vi "Process.vi"(8 "error in":errorcluster, 11 "Instrument.Example":refnum<class "Instrument.Oxford1820.lvclass">) -> (0 "error out":errorcluster, 3 "Instrument.Example out":refnum<class "Instrument.Oxford1820.lvclass">)   [LabVIEW 2019, in "Instrument.Oxford1820.lvclass"]
doc: "---------------------------------------------------------------\nJKI State Machine Objects™\nhttp://jki.net/state-machine-objects/\nCopyright (C) 2005-2015, JKI <info@jki.net>\nALL RIGHTS RESERVED"
uses:
  Instrument.Oxford1820.lvclass
  C:/Program Files/National Instruments/LabVIEW 2019/vi.lib/JKI/JKI SMO/SMO/SMO.lvclass
  C:/Program Files/National Instruments/LabVIEW 2019/user.lib/LevyLab/Instrument Framework/Instrument/Instrument.lvclass
  Typedefs/PrivateEvents--Instrument.Oxford1820.setMagnet.ctl
  <userlib>/LevyLab/Instrument Framework/Instrument Types/Cryostat/Typedefs/Magnet Axis--Enum.ctl
  <userlib>/LevyLab/Instrument Framework/Instrument Types/Cryostat/Typedefs/Magnet Mode--Enum.ctl
  <userlib>/LevyLab/Instrument Framework/Instrument Types/Cryostat/Typedefs/setMagnet--cluster.ctl
  <userlib>/LevyLab/RemoteControl/RemoteControl/Typedefs/Message--Cluster.ctl
  Typedefs/Instrument.Oxford1820.protectedCommands-enum.ctl
  Instrument.Oxford1820.lvclass/Instrument.Oxford1820.ctl
  <vilib>/JKI/JKI SMO/SMO/SMO.lvclass/SMO.ctl
  <instrlib>/Mercury iXX/Public/Libraries/Magnet/Controls/PSU Actions.ctl
  <instrlib>/Mercury iXX/Public/Libraries/Magnet/Controls/Switch Heater.ctl
  Typedefs/Fill Mode-Combo.ctl
  186db9c5-65d2-4fc6-8f89-8e5e62c6db85.vi
  d6eb67ea-c813-4959-b2d5-db01b126de05.vi
  79230e88-dac9-4f3c-b189-792686af81b5.vi
  2ec46187-1f5b-4c8a-9eba-53bd0c375d13.vi
  358ba730-dd62-46a8-9efd-e7dccbf66e54.vi
  c920ba95-1430-4558-8b27-62dbbfd83a50.vi
  <vilib>/dlg_ctls.llb/Space Constant.vi
  <vilib>/AdvancedString/1D String Array to Delimited String.vi
  186db9c5-65d2-4fc6-8f89-8e5e62c6db85.vi/0a7a26e5-3983-4de9-a886-1b2665f625f1.vi
  186db9c5-65d2-4fc6-8f89-8e5e62c6db85.vi/067870e1-bb36-4859-91df-debdbf4baae4.vi
  <vilib>/JKI/JKI SMO/SMO/Private/ReftoDVR--SMO.vi
  d6eb67ea-c813-4959-b2d5-db01b126de05.vi/35af6c41-d28b-4c86-bf85-588a84a7ed82.vi
  d6eb67ea-c813-4959-b2d5-db01b126de05.vi/18926865-8741-4660-bc11-64031fabb0ef.vi
  79230e88-dac9-4f3c-b189-792686af81b5.vi/9a2d704e-5f19-4206-ba54-236c9ffa4be8.vi
  79230e88-dac9-4f3c-b189-792686af81b5.vi/980f9c9d-13e7-4935-b9e6-1304dd0781c0.vi
  2ec46187-1f5b-4c8a-9eba-53bd0c375d13.vi/43f0deac-4eb7-47d7-baca-62a8f74b0a96.vi
  2ec46187-1f5b-4c8a-9eba-53bd0c375d13.vi/e6f40672-4e2f-465c-8f83-0c6010a026af.vi
  358ba730-dd62-46a8-9efd-e7dccbf66e54.vi/002d1415-4ace-441f-9214-6bf758fc91ec.vi
  358ba730-dd62-46a8-9efd-e7dccbf66e54.vi/d6bfcf14-f756-4c59-824c-a5b7ea6121ce.vi
  c920ba95-1430-4558-8b27-62dbbfd83a50.vi/42d7fbcc-e1e5-48c6-b631-238e61f5951c.vi
  c920ba95-1430-4558-8b27-62dbbfd83a50.vi/28ba82e0-a687-457f-9ef5-8b78e327060a.vi
  <vilib>/Utility/Data Type/Get Type Information.vi
  <vilib>/JDP Science/JSONtext/JSON text to Variant.vi
  <userlib>/LevyLab/Instrument Framework/Instrument/API/Instrument.sendMessageToProcess (variant).vi
  <vilib>/JDP Science/JSONtext/LVClass Serializer/JSONtext LVClass Serializer.lvclass
  <userlib>/LevyLab/Instrument Framework/Instrument Types/Cryostat/Instrument.Cryostat.lvclass
  <vilib>/JKI/JKI SMO/SMO/SMO.lvclass
  <instrlib>/Mercury iXX/Public/Libraries/Magnet.lvlib
  <userlib>/LevyLab/RemoteControl/RemoteControl/RemoteControl.lvclass
  <userlib>/LevyLab/Instrument Framework/Instrument/Instrument.lvclass
  <userlib>/LevyLab/Debug/Debug.lvlib
  C:/Program Files/National Instruments/LabVIEW 2019/user.lib/LevyLab/Instrument Framework/Instrument Types/Cryostat/Instrument.Cryostat.lvclass
panel:
  out "Timer":string
  out "State History":string
  out "timer":u32
  # "1820"
  # "1820"
  # "For instructions on how to use the JKI State Machine Objects, examples and video tutorials, visit:\nhttp://jki.net/state-machine-objects/\n\nJKI State Machine Objects™\nhttp://jki.net/state-machine-objects/\nCopyright (C) 2005-2015, JKI <info@jki.net>\nALL RIGHTS RESERVED"
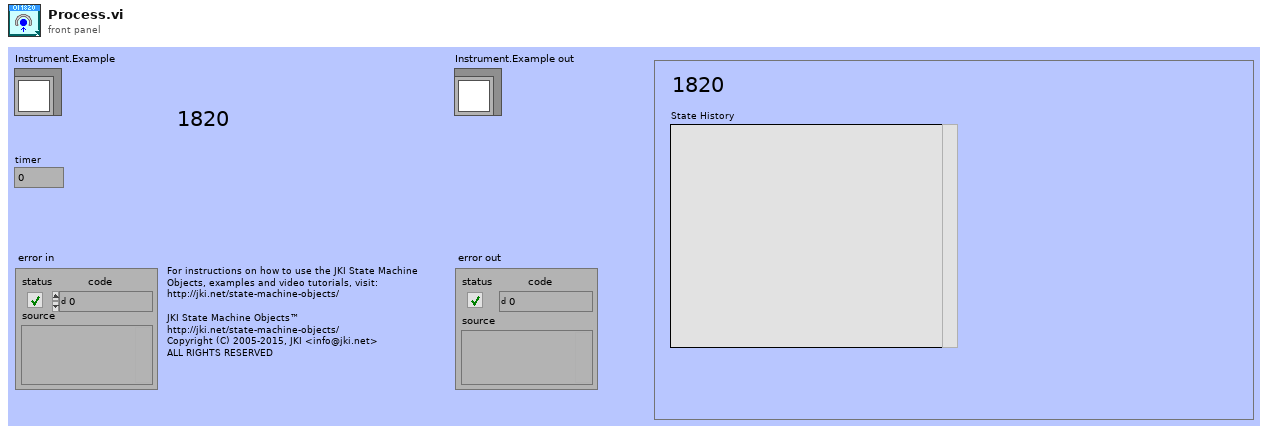
[diagram p1: front panel]
types:
  T1 = typedef "Instrument.Oxford1820.lvclass/PrivateEvents--Instrument.Oxford1820.setMagnet.ctl" = cluster{"field":dbl, "rate":dbl, "axis":T2, "mode":T3}
  T2 = typedef "Instrument.Cryostat.lvclass/Magnet Axis--Enum.ctl" = enum16{"X", "Y", "Z"}
  T3 = typedef "Instrument.Cryostat.lvclass/Magnet Mode--Enum.ctl" = enum16{"Persistent", "Driven"}
  T4 = typedef "Instrument.Cryostat.lvclass/setMagnet--cluster.ctl" = cluster{"field":dbl, "rate":dbl, "axis":T2, "mode":T3}
  T5 = enum32{"invalid app kind", "Development System", "Run Time System", "Student Edition", "Embedded LabVIEW", "Evaluation", "Custom"}
  T6 = typedef "RemoteControl.lvlib/RemoteControl.lvclass/Message--Cluster.ctl" = cluster{"Command":string, "Data":variant, "ID":string, "error":errorcluster}
  T7 = typedef "Instrument.Oxford1820.lvclass/Instrument.Oxford1820.protectedCommands-enum.ctl" = enum16{"Hold", "RampToSet", "RampToZero", "Clamp", "setTarget", "setSwitchHeat", "setLambda", "setFillMode", "setNeedleValve", "getStatus", "getTarget", "getSwitchHeat", "getPSUField", "setSequenceStatus"}
  T8 = enum32{"Invalid", "Standard", "Closed", "Hidden", "Minimized", "Maximized"}
  T9 = typedef "Mercury iXX.lvlib/Magnet.lvlib/PSU Actions.ctl" = string
  T10 = typedef "Mercury iXX.lvlib/Magnet.lvlib/Switch Heater.ctl" = string
  T11 = typedef "Instrument.Oxford1820.lvclass/Fill Mode-Combo.ctl" = string
  T12 = cluster{"Core":cluster{"Current VI Reference":refnum<vi>, "Close Panel on Exit?":bool, "Last Error":cluster{"error":errorcluster, "previous state":string, "remaining states":string}, "Shutdown?":bool}, "SMO":refnum<class "Instrument.Oxford1820.lvclass">, "setMagnet":T4, "Running Step":i32, "sequence":string[], "Message":T6}
  T13 = cluster{"Current VI Reference":refnum<vi>, "Close Panel on Exit?":bool, "Last Error":cluster{"error":errorcluster, "previous state":string, "remaining states":string}, "Shutdown?":bool}
  T14 = typedef "Debug.lvlib/Attribute.Debug.lvclass/DebugBehavior.ctl" = enum16{"Normal", "Debug"}
  T15 = typedef "SMO.lvclass/Protected Events.ctl" = cluster{"StopProcesses":refnum<user-event>, "AbortProcesses":refnum<user-event>, "Config Changed":refnum<user-event>, "Dependency":refnum<user-event>}
  T16 = typedef "Instrument.Oxford1820.lvclass/PrivateEvents--Cluster.ctl" = cluster{"SequenceSetMagnetField":refnum<user-event>, "AbortSequence":refnum<user-event>, "MessageToProcess":refnum<user-event>}
  T17 = typedef "Instrument.Oxford1820.lvclass/getAll.ctl" = cluster{"1820_IPS_Magnet_Field":dbl, "1820_IPS_PS_Field":dbl, "1820_IPS_Target_Field":dbl, "1820_IPS_Target_Field_Rate":dbl, "1820_IPS_Voltage":dbl, "1820_IPS_Current":dbl, "1820_IPS_Level_N2":dbl, "1820_IPS_Level_He":dbl, "1820_IPS_Magnet_Temperature":dbl, "1820_IPS_Magnet_Temperature_R":dbl, "1820_IPS_M1_Current":dbl, "1820_IPS_M1_Voltage":dbl, "1820_IPS_M2_Current":dbl, "1820_IPS_M2_Voltage":dbl, "1820_IPS_M3_Current":dbl, "1820_IPS_M3_Voltage":dbl, "1820_IPS_Status":string, "1820_IPS_Switch":string, "1820_ITC_Lambda_Temperature":dbl, "1820_ITC_Lambda_Temperature_R":dbl, "1820_ITC_Pressure":dbl, "1820_ITC_Needle_Valve":dbl}
  T18 = cluster{"Holding":bool, "Ramp to Setpoint":bool, "Ramp to Zero":bool, "Clamp":bool}
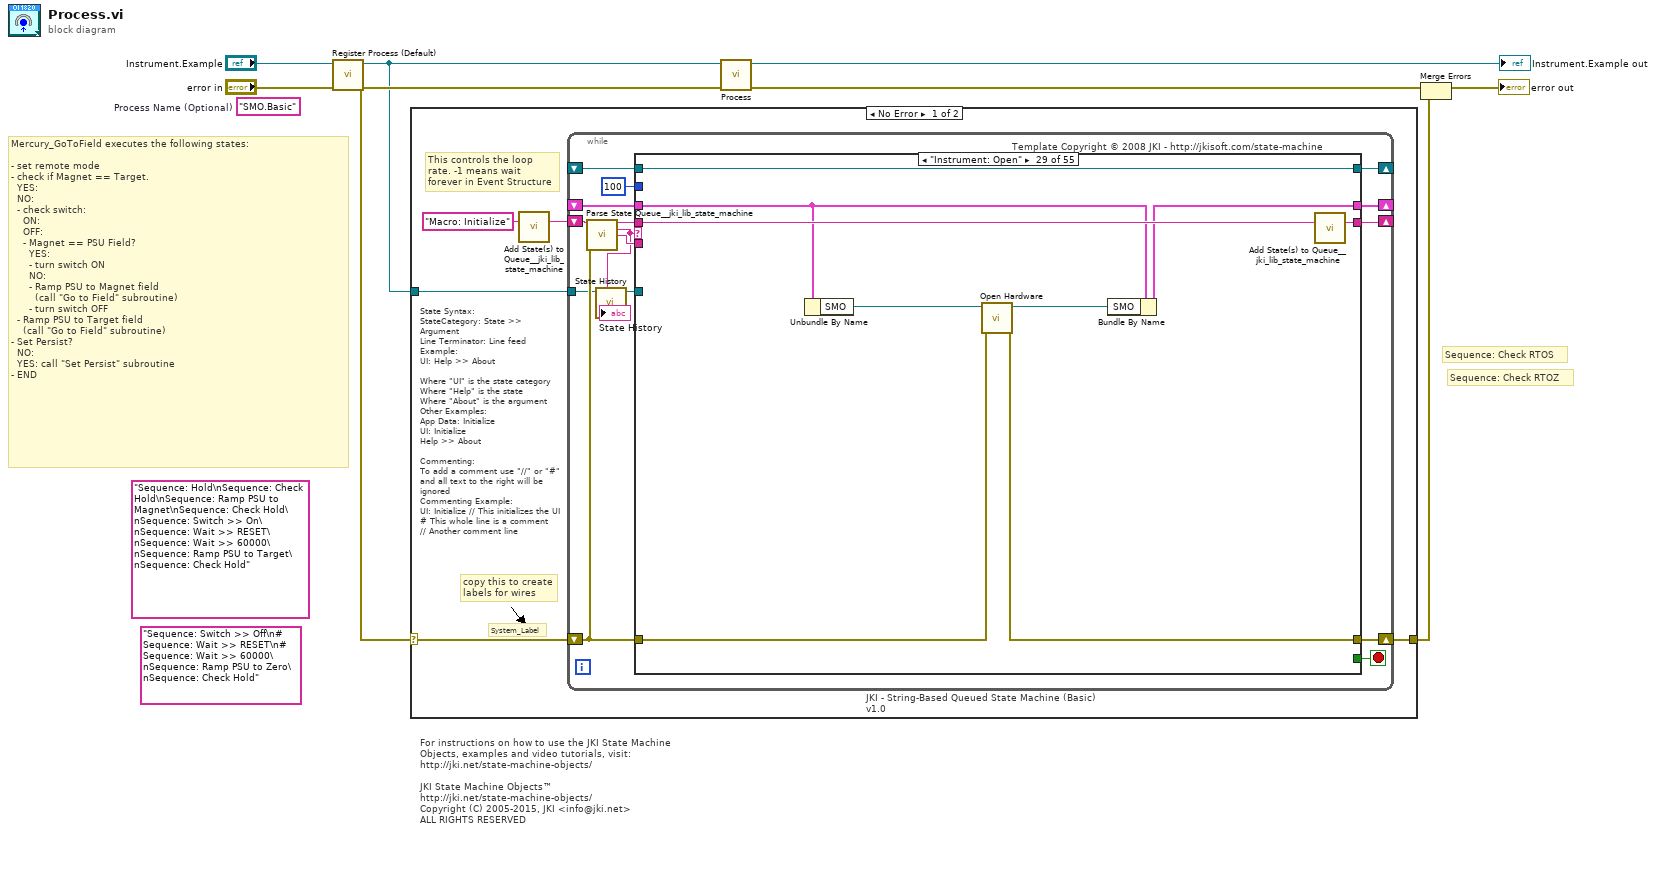
[diagram p0: block diagram]
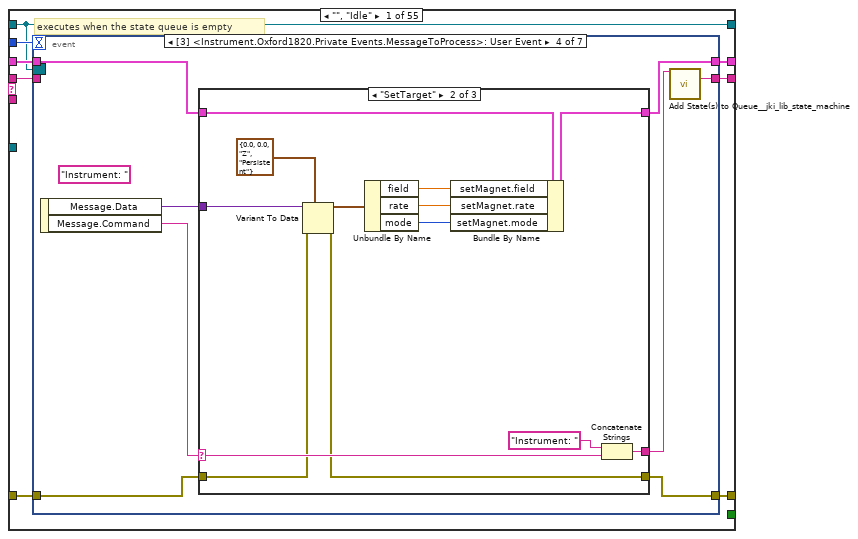
[diagram p2: hidden frame]
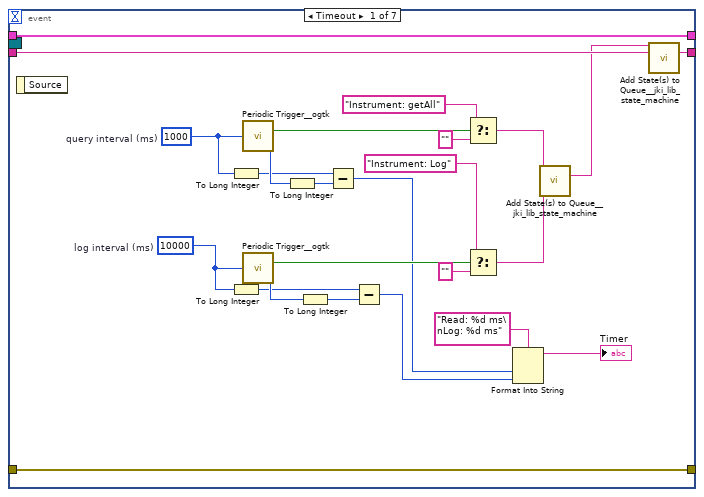
[diagram p3: hidden frame]
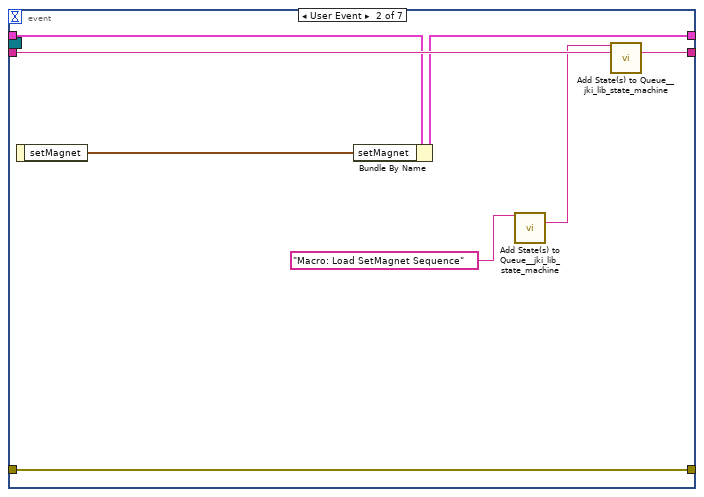
[diagram p4: hidden frame]
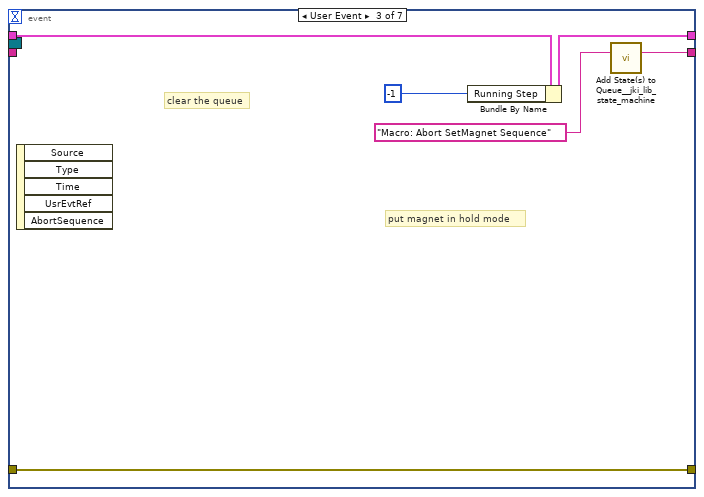
[diagram p5: hidden frame]
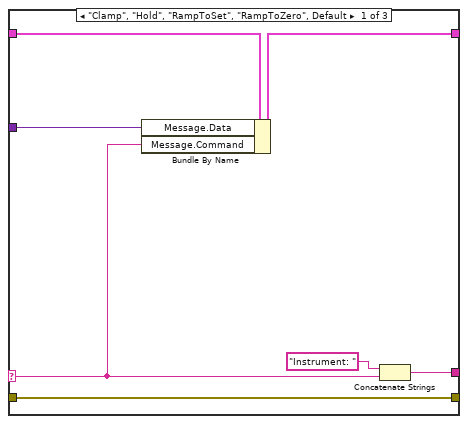
[diagram p6: hidden frame]
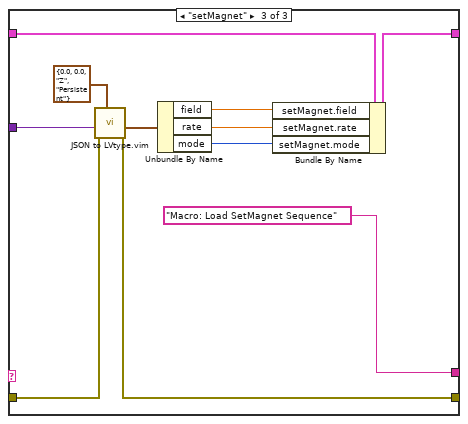
[diagram p7: hidden frame]
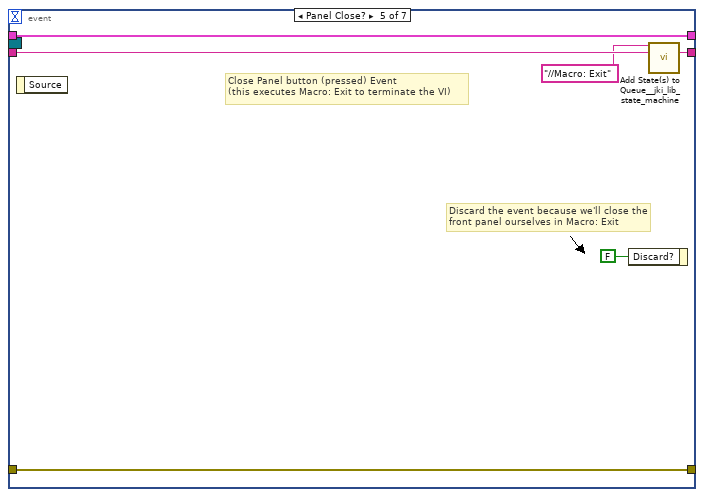
[diagram p8: hidden frame]
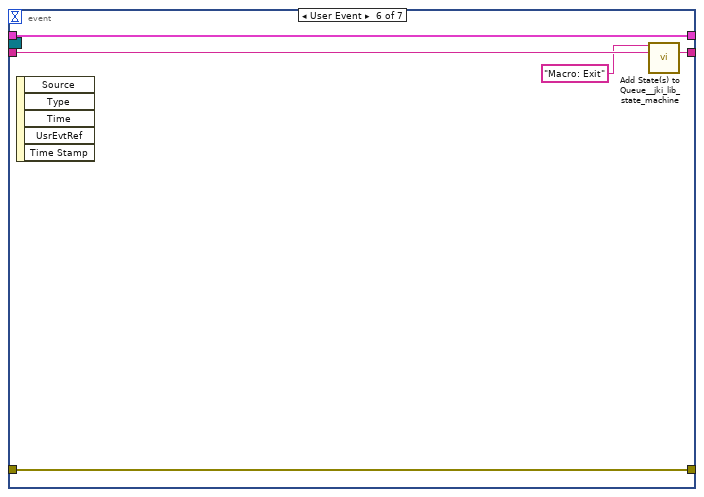
[diagram p9: hidden frame]
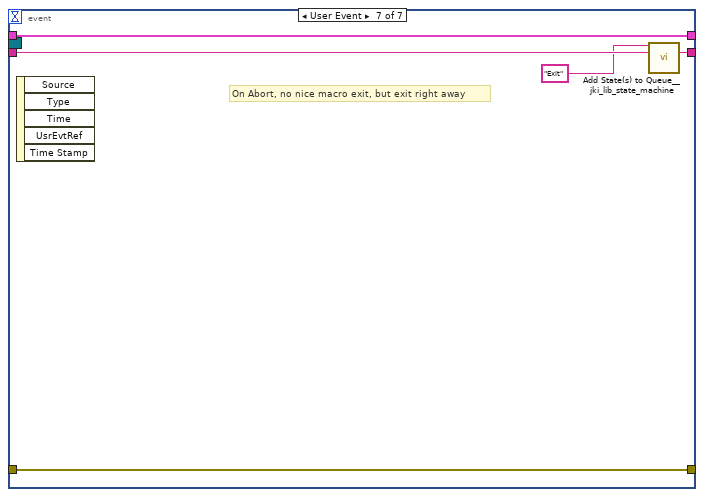
[diagram p10: hidden frame]
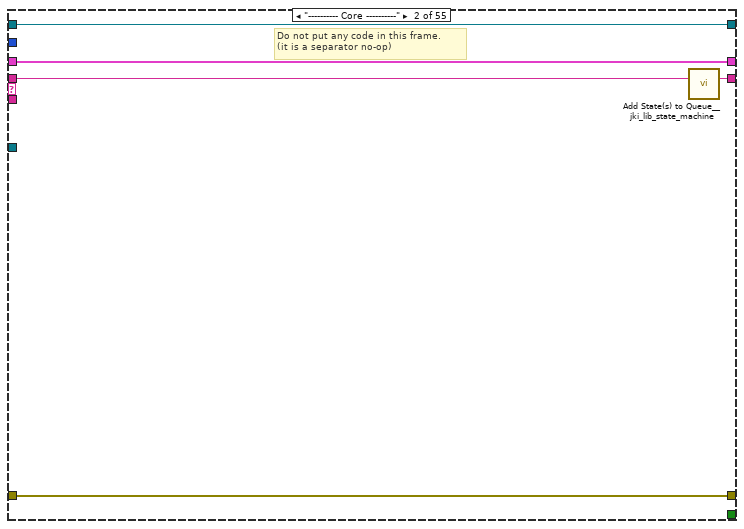
[diagram p11: hidden frame]
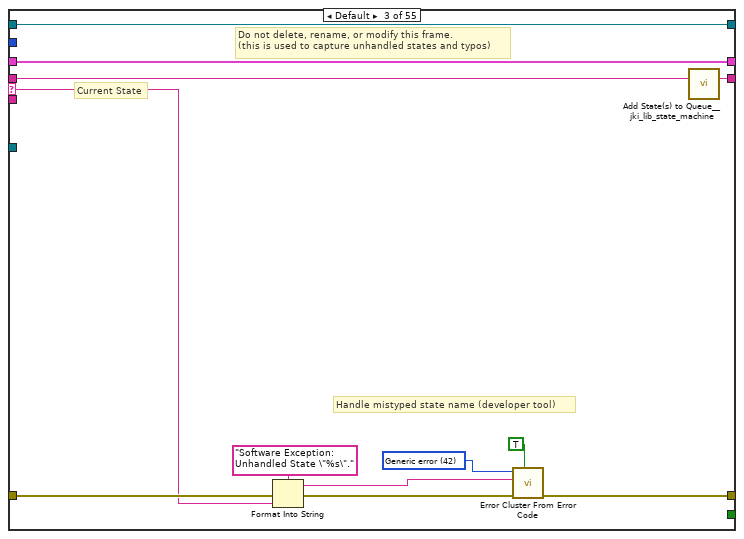
[diagram p12: hidden frame]
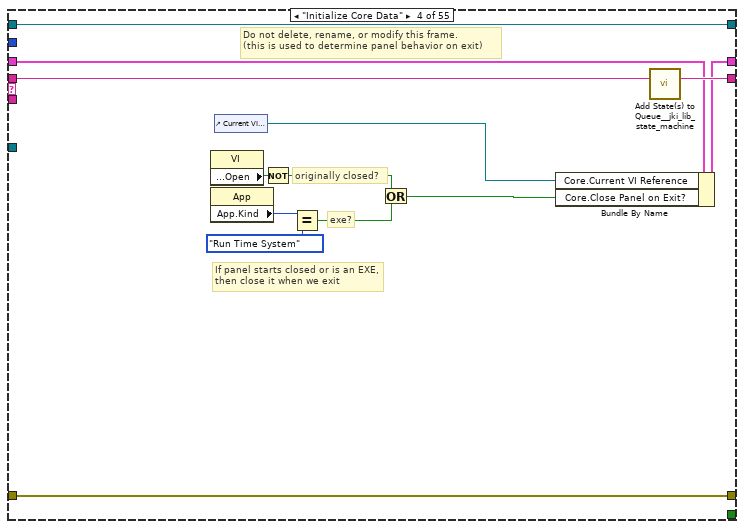
[diagram p13: hidden frame]
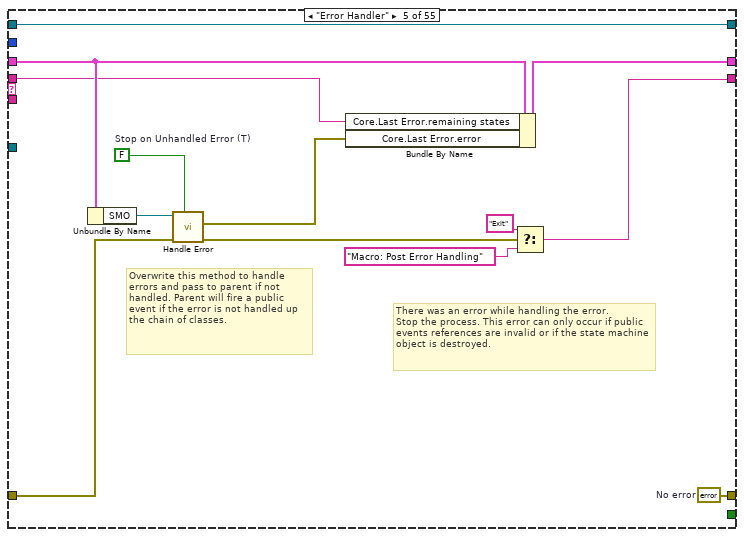
[diagram p14: hidden frame]
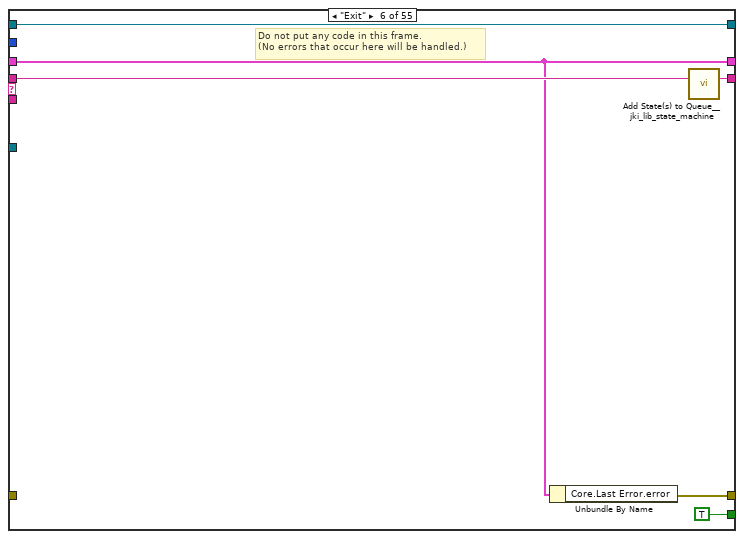
[diagram p15: hidden frame]
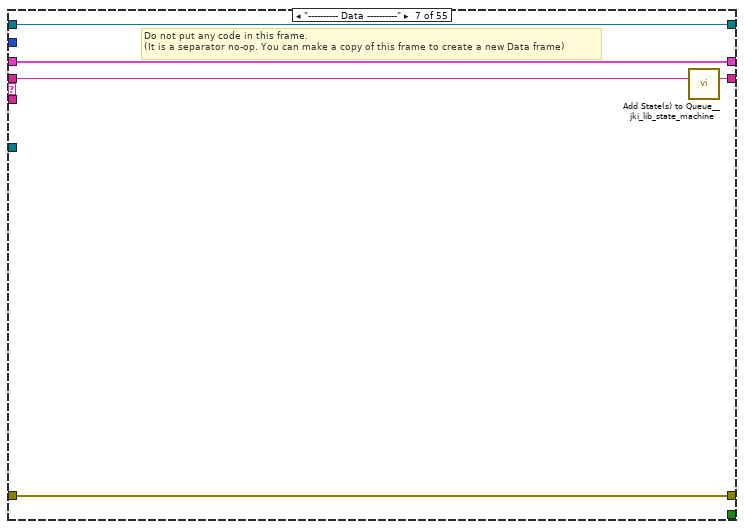
[diagram p16: hidden frame]
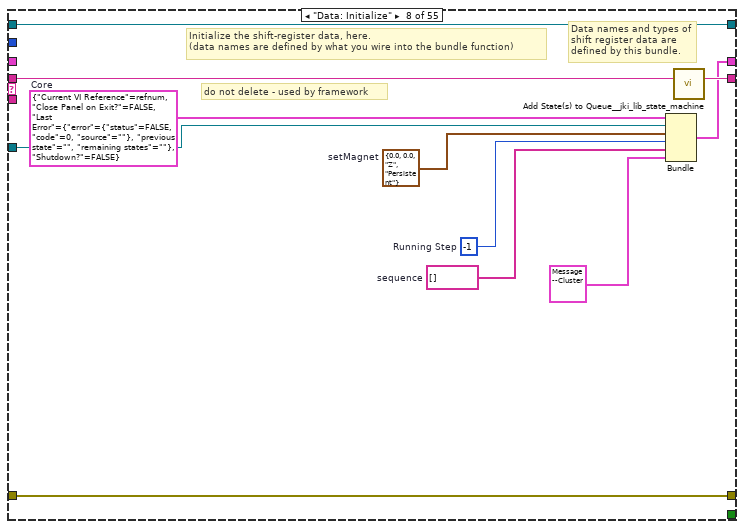
[diagram p17: hidden frame]
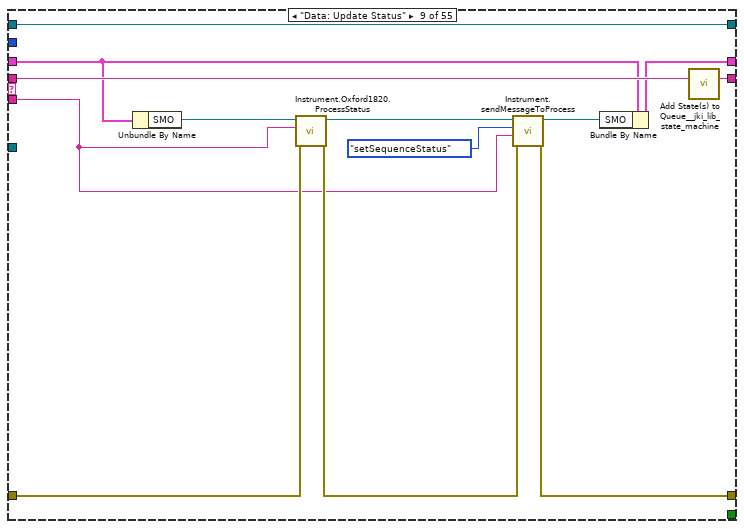
[diagram p18: hidden frame]
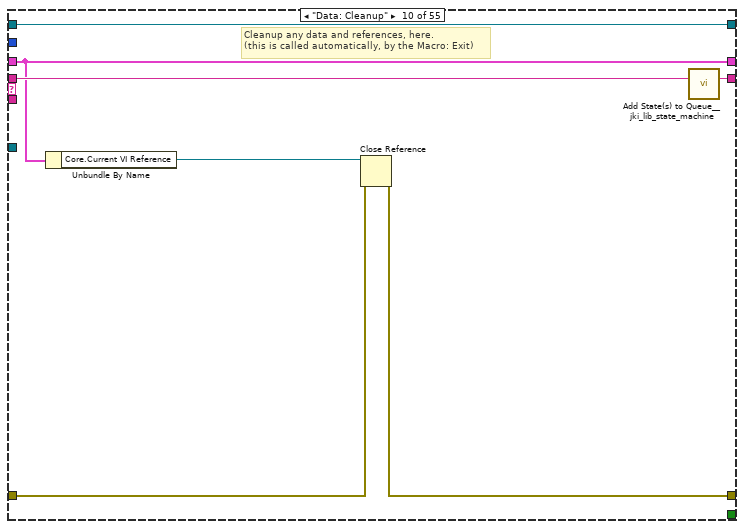
[diagram p19: hidden frame]
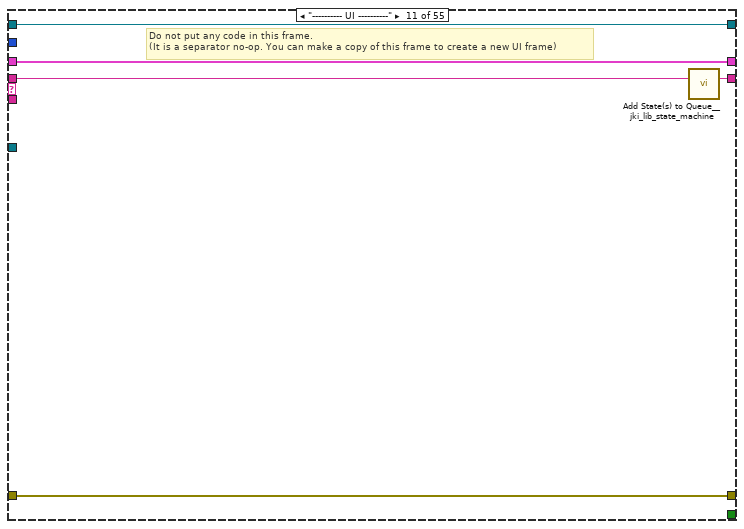
[diagram p20: hidden frame]
diagram:
  (unwired) "Sequence: Switch >> Off\n# Sequence: Wait >> RESET\n# Sequence: Wait >> 60000\nSequence: Ramp PSU to Zero\nSequence: Check Hold" ("State(s) in Front (\"\")")
  (unwired) "Sequence: Hold\nSequence: Check Hold\nSequence: Ramp PSU to Magnet\nSequence: Check Hold\nSequence: Switch >> On\nSequence: Wait >> RESET\nSequence: Wait >> 60000\nSequence: Ramp PSU to Target\nSequence: Check Hold" ("State(s) in Front (\"\")")
  (unwired) "SMO.Basic"  # Process Name (Optional)
  # "Sequence: Check RTOZ"
  # "Sequence: Check RTOS"
  # "Mercury_GoToField executes the following states:\n\n- set remote mode\n- check if Magnet == Target.\n  YES:\n  NO:\n  - check switch:\n    ON:\n    OFF:\n    - Magnet == PSU Field?\n      YES:\n      - turn switch ON\n      NO:\n      - Ramp PSU to Magnet field\n        (call \"Go to Field\" subroutine)\n      - turn switch OFF\n  - Ramp PSU to Target field\n    (call \"Go to Field\" subroutine)\n- Set Persist?\n  NO:\n  YES: call \"Set Persist\" subroutine\n- END"
  # "For instructions on how to use the JKI State Machine Objects, examples and video tutorials, visit:\nhttp://jki.net/state-machine-objects/\n\nJKI State Machine Objects™\nhttp://jki.net/state-machine-objects/\nCopyright (C) 2005-2015, JKI <info@jki.net>\nALL RIGHTS RESERVED"
  n1 = call <vilib>:"Register Process (Default).vi"("error in (no error)"="error in", "SMO"="Instrument.Example") -> ("error out"=w5:errorcluster, "SelfRef"=w4:refnum<class "Instrument.Oxford1820.lvclass">)  [unwired: 8 in]
  n2 = case shown="No Error" w5 {
    selector: w5 -> [w10 w914]
    tunnel: w4 -> [w11 _]
    tunnel: [w9 w914] -> w1
    frame No Error {
      # "State Syntax:\nStateCategory: State >> Argument\nLine Terminator: Line feed\nExample:\nUI: Help >> About\n\nWhere \"UI\" is the state category\nWhere \"Help\" is the state\nWhere \"About\" is the argument\nOther Examples:\nApp Data: Initialize\nUI: Initialize\nHelp >> About\n\nCommenting:\nTo add a comment use \"//\" or \"#\" and all text to the right will be ignored\nCommenting Example:\nUI: Initialize // This initializes the UI\n# This whole line is a comment\n// Another comment line"
      # "copy this to create labels for wires"
      # "This controls the loop rate. -1 means wait forever in Event Structure"
      # "System_Label"
      n3 = call <vilib>:"Add State(s) to Queue__jki_lib_state_machine.vi"("State(s) in (\"\")"="Macro: Initialize") -> ("States Out"=w13:string)  [unwired: 14 in]
      n4 = while "JKI - String-Based Queued State Machine (Basic) v1.0" {
        shift-right: [w23] -> _
        shift-left: _ -> [w22]
        shift-right: [w26] -> w9
        shift-left: w10 -> [w20]
        shift-right: [w25] -> _
        shift-left: w13 -> [w27]
        tunnel: w11 -> [w14]
        shift-right: [w19] -> _
        shift-left: _ -> [w18]
        stop <- w24 stop-if-true
        # "Template Copyright © 2008 JKI - http://jkisoft.com/state-machine"
        n5 = call <vilib>:"Parse State Queue__jki_lib_state_machine.vi"("State Queue"=w27, "Error In (no error)"=w20) -> ("Remaining States"=w29:string, "Current State"=w16:string, "Arguments"=w28:string)  [unwired: 11 in]
        n6 = call <userlib>:"State History.vi"("Current State"=w16, "SMO"=w14) -> ("SMO"=w15:refnum<class "Instrument.Oxford1820.lvclass">, "History"=→"State History":string)  [unwired: 8 in]
        n7 = case shown="\"Instrument: Open\"" w16 {
          selector: w16 -> [_ _ w138 _ _ _ _ _ _ _ _ _ _ _ _ _ _ _ _ _ _ _ _ _ _ _ _ _ _ _ _ _ _ _ _ _ _ _ _ _ _ _ _ _ _ w687 w711 w744 w776 w797 w817 w837 w858 w877 w904]
          tunnel: w29 -> [w37 w136 w142 w161 w163 w180 w185 w196 w209 w216 w221 w228 w235 w251 w283 w292 w309 w324 w346 w349 _ _ w405 w416 w421 w434 w440 w447 w456 w465 w477 w490 w503 w520 w533 w550 w560 w573 w598 w618 w631 w644 w653 w662 w684 w696 w717 w750 w782 w804 w825 w846 w867 w888 w913]
          tunnel: w28 -> [_ _ _ _ _ _ _ _ w197 _ _ _ w229 w245 _ _ _ _ _ _ _ _ _ _ _ _ _ _ _ _ _ _ w493 _ _ _ _ w565 w584 _ _ _ _ _ w668 _ w710 _ _ _ _ _ _ _ _]
          tunnel: w22 -> [w35 w133 w140 w152 w170 w176 w182 _ w206 w211 w218 w226 w233 w247 w280 w289 w293 w311 w335 w350 w366 w393 w402 w413 w418 w432 w438 w442 w452 w461 w474 w487 w496 w515 w526 w545 w555 w562 w594 w614 w627 w640 w649 w656 w671 w693 w714 w746 w779 w801 w819 w840 w861 w885 w910]
          tunnel: [w34 w134 w144 w158 w171 w175 w183 w187 w198 w212 w219 w222 w230 w248 w281 w284 w307 w314 w344 w351 w367 w391 w403 w407 w419 w427 w436 w444 w448 w457 w467 w478 w491 w511 w527 w542 w551 w563 w588 w608 w622 w637 w647 w659 w672 w689 w698 w735 w769 w795 w811 w831 w852 w872 w903] -> w26
          tunnel: w20 -> [w33 w134 w143 w158 w172 _ w183 w187 w204 w213 w219 w223 w231 w249 w281 w284 w307 w313 w344 w351 w367 w391 w403 w408 w419 w428 w436 w444 w449 w458 w472 w479 w494 w513 w525 w543 w553 w566 w585 w606 w619 w633 w646 w659 w669 w689 w697 w734 w768 w795 w805 w826 w847 w868 w889]
          tunnel: [w36 w135 w141 w160 w162 w179 w184 w195 w208 w215 w220 w227 w234 w250 w282 w291 w308 w323 w345 w348 w383 w400 w404 w415 w420 w433 w439 w446 w455 w464 w476 w489 w502 w519 w532 w549 w559 w572 w597 w617 w630 w643 w652 w661 w683 w695 w716 w749 w781 w803 w824 w845 w866 w887 w912] -> w25
          tunnel: [_ _ _ _ _ TRUE _ _ _ _ _ _ _ _ _ _ _ _ _ _ _ _ _ _ _ _ _ _ _ _ _ _ _ _ _ _ _ _ _ _ _ _ _ _ _ _ _ _ _ _ _ _ _ _ _] -> w24
          tunnel: [w32 w133 w140 w159 w169 w176 w182 w194 w203 w211 w218 w226 w233 w247 w280 w289 w294 w312 w342 w347 w375 w395 w402 w413 w418 w432 w438 w441 w450 w459 w473 w486 w500 w517 w530 w547 w557 w570 w595 w615 w628 w641 w650 w655 w665 w692 w713 w745 w778 w800 w818 w839 w860 w884 w909] -> w23
          tunnel: 100 ("Timeout") -> [w31 _ _ _ _ _ _ _ _ _ _ _ _ _ _ _ _ _ _ _ _ _ _ _ _ _ _ _ _ _ _ _ _ _ _ _ _ _ _ _ _ _ _ _ _ _ _ _ _ _ _ _ _ _ _]
          tunnel: w15 -> [_ _ _ _ _ _ _ w188 _ _ _ _ _ _ _ _ _ _ _ _ _ _ _ _ _ _ _ _ _ _ _ _ _ _ _ _ _ _ _ _ _ _ _ _ _ _ _ _ _ _ _ _ _ _ _]
          tunnel: [w30 w132 w137 w149 w174 w177 w181 w193 w207 w210 w217 w225 w232 w244 w279 w290 w301 w322 w343 w358 w382 w399 w401 w414 w417 w431 w437 w445 w454 w463 w475 w488 w501 w518 w531 w548 w558 w571 w596 w616 w629 w642 w651 w660 w682 w694 w715 w748 w780 w802 w823 w844 w865 w886 w911] -> w19
          tunnel: w18 -> [w30 w132 w137 w149 w174 w177 w181 w193 w207 w210 w217 w225 w232 w244 w279 w290 w301 w322 w343 w358 w382 w399 w401 w414 w417 _ w437 w445 w454 w463 w475 w488 w501 w518 w531 w548 w558 w571 w596 w616 w629 w642 w651 w660 w682 w694 w715 w748 w780 w802 w823 w844 w865 w886 w911]
          frame "", "Idle" {
            # "executes when the state queue is empty"
            n8 = event shown="[3] <Instrument.Oxford1820.Private Events.MessageToProcess>: User Event" {
              selector: w30 -> [_ _ _ _ _ _ _]
              dyn-events: _ -> [_ _ _ _ _ _ _]
              timeout: w31 -> [_ _ _ _ _ _ _]
              tunnel: w37 -> [w62 w68 _ _ w121 w126 w131]
              tunnel: [w61 w69 w75 w84 w120 w125 w130] -> w36
              tunnel: w35 -> [w59 w67 w73 w79 w118 w123 w128]
              tunnel: [w60 w70 w76 w83 w119 w124 w129] -> w34
              tunnel: w33 -> [w60 w70 w76 w82 w119 w124 w129]
              tunnel: [w59 w66 w72 w78 w118 w123 w128] -> w32
              event Timeout {
                w38 = u32 10000  # log interval (ms)
                w39 = u32 1000  # query interval (ms)
                n9 = event-data() -> ()  [unwired: 1 in, 1 out]
                n10 = To Long Integer(number=w39) -> (32bit integer=w45:i32)
                n11 = To Long Integer(number=w38) -> (32bit integer=w46:i32)
                n12 = call <userlib>:"Periodic Trigger__ogtk.vi"("time (ms)"=w39) -> ("Triggered"=w58:bool, "timer value"=w52:u32)  [unwired: 12 in, 1 out]
                n13 = call <userlib>:"Periodic Trigger__ogtk.vi"("time (ms)"=w38) -> ("Triggered"=w55:bool, "timer value"=w51:u32)  [unwired: 12 in, 1 out]
                n14 = To Long Integer(number=w52) -> (32bit integer=w44:i32)
                n15 = To Long Integer(number=w51) -> (32bit integer=w43:i32)
                n16 = Subtract(x=w45, y=w44) -> (x-y=w50:i32)
                n17 = Subtract(x=w46, y=w43) -> (x-y=w49:i32)
                n18 = Select(t="Instrument: getAll", s=w58, f="") -> (s? t:f=w53:string)
                n19 = Select(t="Instrument: Log", s=w55, f="") -> (s? t:f=w54:string)
                n20 = Format Into String(format string="Read: %d ms\nLog: %d ms", w50, w49) -> (resulting string=→"Timer":string)  [unwired: 2 in, 1 out]
                n21 = call <vilib>:"Add State(s) to Queue__jki_lib_state_machine.vi"("State(s) in Front (\"\")"=w53, "State(s) at Back (\"\")"=w54) -> ("States Out"=w40:string)  [unwired: 13 in]
                n22 = call <vilib>:"Add State(s) to Queue__jki_lib_state_machine.vi"("State(s) in Front (\"\")"=w40, "State(s) in (\"\")"=w62) -> ("States Out"=w61:string)  [unwired: 13 in]
              }
              event User Event {
                n23 = event-data() -> ("setMagnet"=w63:T4)  [unwired: 1 in]
                n24 = Bundle By Name(cluster=w67, "setMagnet"=w63) -> (w66:T12)
                n25 = call <vilib>:"Add State(s) to Queue__jki_lib_state_machine.vi"("State(s) in Front (\"\")"="Macro: Load SetMagnet Sequence" ("State(s) at Back (\"\")")) -> ("States Out"=w64:string)  [unwired: 14 in]
                n26 = call <vilib>:"Add State(s) to Queue__jki_lib_state_machine.vi"("State(s) in Front (\"\")"=w64, "State(s) in (\"\")"=w68) -> ("States Out"=w69:string)  [unwired: 13 in]
              }
              event User Event {
                # "put magnet in hold mode"
                # "clear the queue"
                n27 = event-data() -> ()  [unwired: 1 in, 5 out]
                n28 = Bundle By Name(cluster=w73, "Running Step"=-1) -> (w72:T12)
                n29 = call <vilib>:"Add State(s) to Queue__jki_lib_state_machine.vi"("State(s) in (\"\")"="Macro: Abort SetMagnet Sequence" ("State(s) at Back (\"\")")) -> ("States Out"=w75:string)  [unwired: 14 in]
              }
              event User Event {
                (unwired) "Instrument: " ("State(s) at Back (\"\")")
                n30 = event-data() -> ("Message.Data"=w80:variant, "Message.Command"=w81:string)  [unwired: 1 in]
                n31 = case shown="\"SetTarget\"" w81 {
                  selector: w81 -> [w87 w103 _]
                  tunnel: w79 -> [w85 w101 w115]
                  tunnel: [w86 w100 w114] -> w78
                  tunnel: [w91 w104 "Macro: Load SetMagnet Sequence" ("State(s) at Back (\"\")")] -> w77
                  tunnel: w80 -> [w88 w99 w109]
                  tunnel: w82 -> [w89 w97 w106]
                  tunnel: [w89 w96 w105] -> w83
                  frame "Clamp", "Hold", "RampToSet", "RampToZero", Default {
                    n32 = Bundle By Name(cluster=w85, "Message.Data"=w88, "Message.Command"=w87) -> (w86:T12)
                    n33 = Concatenate Strings("Instrument: " ("State"), w87) -> (w91:string)
                  }
                  frame "SetTarget" {
                    n34 = Variant To Data(error in=w97, type=T1 {"field"=0.0, "rate"=0.0, "axis"=enum."Z", "mode"=enum."Persistent"} ("Set Magnet Field"), Variant=w99) -> (data=w95:T1, error out=w96:errorcluster)
                    n35 = Unbundle By Name(w95) -> ("field"=w94:dbl, "rate"=w98:dbl, "mode"=w92:T3)
                    n36 = Bundle By Name(cluster=w101, "setMagnet.field"=w94, "setMagnet.rate"=w98, "setMagnet.mode"=w92) -> (w100:T12)
                    n37 = Concatenate Strings("Instrument: " ("State"), w103) -> (w104:string)
                  }
                  frame "setMagnet" {
                    n38 = call "JSON to LVtype.vim"("type"=T4 {"field"=0.0, "rate"=0.0, "axis"=enum."Z", "mode"=enum."Persistent"} ("setMagnet"), "error in (no error)"=w106, "JSON Data in"=w109) -> ("error out"=w105:errorcluster, "Data out"=w107:T4)  [unwired: 7 in]
                    n39 = Unbundle By Name(w107) -> ("field"=w110:dbl, "rate"=w111:dbl, "mode"=w112:T3)
                    n40 = Bundle By Name(cluster=w115, "setMagnet.field"=w110, "setMagnet.rate"=w111, "setMagnet.mode"=w112) -> (w114:T12)
                  }
                }
                n41 = call <vilib>:"Add State(s) to Queue__jki_lib_state_machine.vi"("State(s) in Front (\"\")"=w77) -> ("States Out"=w84:string)  [unwired: 14 in]
              }
              event Panel Close? {
                # "Discard the event because we'll close the front panel ourselves in Macro: Exit"
                # "Close Panel button (pressed) Event\n(this executes Macro: Exit to terminate the VI)"
                n42 = event-data() -> ()  [unwired: 1 in, 1 out]
                n43 = event-data("Discard?"=FALSE) -> ()  [unwired: 1 in, 1 out]
                n44 = call <vilib>:"Add State(s) to Queue__jki_lib_state_machine.vi"("State(s) in Front (\"\")"="//Macro: Exit", "State(s) in (\"\")"=w121) -> ("States Out"=w120:string)  [unwired: 13 in]
              }
              event User Event {
                n45 = event-data() -> ()  [unwired: 1 in, 5 out]
                n46 = call <vilib>:"Add State(s) to Queue__jki_lib_state_machine.vi"("State(s) in Front (\"\")"="Macro: Exit", "State(s) in (\"\")"=w126) -> ("States Out"=w125:string)  [unwired: 13 in]
              }
              event User Event {
                # "On Abort, no nice macro exit, but exit right away"
                n47 = event-data() -> ()  [unwired: 1 in, 5 out]
                n48 = call <vilib>:"Add State(s) to Queue__jki_lib_state_machine.vi"("State(s) in Front (\"\")"="Exit", "State(s) in (\"\")"=w131) -> ("States Out"=w130:string)  [unwired: 13 in]
              }
            }
          }
          frame "---------- Core ----------" {
            # "Do not put any code in this frame.\n(it is a separator no-op)"
            n49 = call <vilib>:"Add State(s) to Queue__jki_lib_state_machine.vi"("State(s) in (\"\")"=w136) -> ("States Out"=w135:string)  [unwired: 14 in]
          }
          frame Default {
            w147 = 42 items=["No error", "Argument error", "Memory is full", "Out of zone", "End of file", "File already open", "Generic file I/O error", "File not found", "File permission error", "Disk is full", "Duplicate path", "Too many files open", "System feature not enabled", "Resource file not found", "Cannot add resource", "Resource not found", "Image not found", "Image memory error", "Pen does not exist", "Config type invalid", "Config token not found", "Config parse error", "Config memory error", "Bad external code format", "Bad external code offset", "External code not present", "Null window", "Destroy window error", "Null menu", "Print aborted", "Bad print record", "Print driver error", "Windows error during printing", "Memory error during printing", "Print dialog error", "Generic print error", "Invalid device refnum", "Device not found", "Device parameter error", "Device unit error", "Cannot open device", "Device call aborted", "Generic error", "Cancelled by user", "Object ID too low", "Object ID too high", "Object not in heap", "Unknown heap", "Unknown object (invalid DefProc)", "Unknown object (DefProc not in table)", "Message out of range", "Invalid (null) method", "Unknown message", "Manager call not supported", "Bad address", "Network operation in progress", "Network operation timed out", "Connection is busy", "Network attribute not supported", "Network error", "Address in use", "System out of memory", "Connection aborted", "Connection refused", "Not connected", "Already connected", "Connection closed", "Initialization error (interapplication manager)", "Bad occurrence", "Wait on unbound occurrence handler", "Occurrence queue overflow", "Datalog type conflict", "Unused", "Unrecognized type (interapplication manager)", "Memory corrupt", "Failed to make temporary DLL", "Old CIN version", "Drag socket not found", "Failed to load drop-object", "Failed to register OLE object", "Failed to release OLE object", "Format specifier type mismatch", "Unknown format specifier", "Too few format specifiers", "Too many format specifiers", "Scan failed", "Newer CIN version", "Error converting to variant", "Runtime menu error", "Password tampered", "Variant attribute not found", "Incompatible variant data type", "Event data is not available", "Event Store is not present", "Occurrence is not found", "Event Queue is not created", "Event info is not available", "Refnum passed is NULL", "Error retrieving Class GUID", "Error retrieving CoClass GUID", "Error retrieving TypeLib GUID.", "Bad built application magic bytes.", "Specific driver is different from the specific driver associated with the Logical Name.", "There is no session opened to the class driver.", "Max Error", "MAX - Error with config objects", "MAX - Error loading configuration", "MAX - Group not supported"]
            # "Current State"
            # "Do not delete, rename, or modify this frame.\n(this is used to capture unhandled states and typos)"
            # "Handle mistyped state name (developer tool)"
            n50 = Format Into String(format string="Software Exception: Unhandled State \"%s\"." ("message"), error in=w143, w138) -> (resulting string=w146:string, error out=w145:errorcluster)  [unwired: 1 in]
            n51 = call <vilib>:"Error Cluster From Error Code.vi"("show call chain? (False)"=TRUE, "error in (no error)"=w145, "error message (\"\")"=w146, "error code (0)"=w147) -> ("error out"=w144:errorcluster)  [unwired: 5 in]
            n52 = call <vilib>:"Add State(s) to Queue__jki_lib_state_machine.vi"("State(s) in (\"\")"=w142) -> ("States Out"=w141:string)  [unwired: 14 in]
          }
          frame "Initialize Core Data" {
            # "Do not delete, rename, or modify this frame.\n(this is used to determine panel behavior on exit)"
            # "originally closed?"
            # "exe?"
            # "If panel starts closed or is an EXE, then close it when we exit"
            n53 = property class="VI"() -> ("Front Panel.Open"=w157:bool)  [unwired: 2 in, 2 out]
            n54 = property class="App"() -> ("App.Kind"=w156:T5)  [unwired: 2 in, 2 out]
            n55 = control-ref of="Current VI Reference"() -> (w150:refnum<vi>)
            n56 = Not(x=w157) -> (.not. x?=w154:bool)
            n57 = Equal?(x=w156, y=T5."Run Time System" ("Application:Kind")) -> (x = y?=w153:bool)
            n58 = Or(x=w154, y=w153) -> (x .or. y?=w151:bool)
            n59 = Bundle By Name(cluster=w152, "Core.Current VI Reference"=w150, "Core.Close Panel on Exit?"=w151) -> (w159:T12)
            n60 = call <vilib>:"Add State(s) to Queue__jki_lib_state_machine.vi"("State(s) in (\"\")"=w161) -> ("States Out"=w160:string)  [unwired: 14 in]
          }
          frame "Error Handler" {
            w165 = FALSE  # Stop on Unhandled Error (T)
            w171 = errorcluster {"status"=FALSE, "code"=0, "source"=""}  # No error
            # "There was an error while handling the error.\nStop the process. This error can only occur if public events references are invalid or if the state machine object is destroyed."
            # "Overwrite this method to handle errors and pass to parent if not handled. Parent will fire a public event if the error is not handled up the chain of classes."
            n61 = Unbundle By Name(w170) -> ("SMO"=w173:refnum<class "Instrument.Oxford1820.lvclass">)
            n62 = call-dynamic "Handle Error.vi"("Stop on Unhandled Error (T)"=w165, "error in"=w172, "SMO"=w173) -> ("handling error"=w166:errorcluster, "Unhandled error"=w168:errorcluster)  [unwired: 6 in, 1 out]
            n63 = Bundle By Name(cluster=w170, "Core.Last Error.remaining states"=w163, "Core.Last Error.error"=w168) -> (w169:T12)
            n64 = Select(t="Exit", s=w166, f="Macro: Post Error Handling") -> (s? t:f=w162:string)
          }
          frame "Exit" {
            # "Do not put any code in this frame.\n(No errors that occur here will be handled.)"
            n65 = Unbundle By Name(w176) -> ("Core.Last Error.error"=w175:errorcluster)
            n66 = call <vilib>:"Add State(s) to Queue__jki_lib_state_machine.vi"("State(s) in (\"\")"=w180) -> ("States Out"=w179:string)  [unwired: 14 in]
          }
          frame "---------- Data ----------" {
            # "Do not put any code in this frame.\n(It is a separator no-op. You can make a copy of this frame to create a new Data frame)"
            n67 = call <vilib>:"Add State(s) to Queue__jki_lib_state_machine.vi"("State(s) in (\"\")"=w185) -> ("States Out"=w184:string)  [unwired: 14 in]
          }
          frame "Data: Initialize" {
            w186 = T4 {"field"=0.0, "rate"=0.0, "axis"=enum."Z", "mode"=enum."Persistent"}  # setMagnet
            w190 = string[] []  # sequence
            w191 = -1  # Running Step
            w192 = T13 {"Current VI Reference"=refnum, "Close Panel on Exit?"=FALSE, "Last Error"={"error"={"status"=FALSE, "code"=0, "source"=""}, "previous state"="", "remaining states"=""}, "Shutdown?"=FALSE}  # Core
            # "do not delete - used by framework"
            # "Data names and types of shift register data are defined by this bundle."
            # "Initialize the shift-register data, here.\n(data names are defined by what you wire into the bundle function)"
            n68 = Bundle("Core"=w192, "SMO"=w188, "setMagnet"=w186, "Running Step"=w191, "sequence"=w190, "Message"=T6 {"Command"="", "Data"=variant(string ""), "ID"="", "error"={"status"=FALSE, "code"=0, "source"=""}}) -> (w194:T12)  [unwired: 1 in]
            n69 = call <vilib>:"Add State(s) to Queue__jki_lib_state_machine.vi"("State(s) in (\"\")"=w196) -> ("States Out"=w195:string)  [unwired: 14 in]
          }
          frame "Data: Update Status" {
            n70 = Unbundle By Name(w206) -> ("SMO"=w205:refnum<class "Instrument.Oxford1820.lvclass">)
            n71 = call "Instrument.Oxford1820.ProcessStatus.vi"("error in (no error)"=w204, "event data"=w197, "Instrument.Oxford1820"=w205) -> ("error out"=w199:errorcluster, "Instrument.Oxford1820 out"=w202:refnum<class "Instrument.Oxford1820.lvclass">)  [unwired: 7 in]
            n72 = call-poly <userlib>:"Instrument.sendMessageToProcess.vi"("error in (no error)"=w199, "Data"=w197, "Command"=Instrument.Oxford1820.protectedCommands-enum."setSequenceStatus" ("protectedCommands"), "Instrument"=w202) -> ("error out"=w198:errorcluster, "Instrument out"=w201:refnum<class "Instrument.Oxford1820.lvclass">)  [unwired: 6 in]
            n73 = Bundle By Name(cluster=w206, "SMO"=w201) -> (w203:T12)
            n74 = call <vilib>:"Add State(s) to Queue__jki_lib_state_machine.vi"("State(s) in (\"\")"=w209) -> ("States Out"=w208:string)  [unwired: 14 in]
          }
          frame "Data: Cleanup" {
            # "Cleanup any data and references, here.\n(this is called automatically, by the Macro: Exit)"
            n75 = Unbundle By Name(w211) -> ("Core.Current VI Reference"=w214:refnum<vi>)
            n76 = Close Reference(reference=w214, error in (no error)=w213) -> (error out=w212:errorcluster)
            n77 = call <vilib>:"Add State(s) to Queue__jki_lib_state_machine.vi"("State(s) in (\"\")"=w216) -> ("States Out"=w215:string)  [unwired: 14 in]
          }
          frame "---------- UI ----------" {
            # "Do not put any code in this frame.\n(It is a separator no-op. You can make a copy of this frame to create a new UI frame)"
            n78 = call <vilib>:"Add State(s) to Queue__jki_lib_state_machine.vi"("State(s) in (\"\")"=w221) -> ("States Out"=w220:string)  [unwired: 14 in]
          }
          frame "UI: Initialize" {
            # "Initialize the User Interface, here.\n(this is called automatically, by the Macro: Init)"
            n79 = call <userlib>:"Fit VI window to Largest Dec__ogtk.vi"("error in (no error)"=w223, "border spacing (2 px)"=0) -> ("error out"=w222:errorcluster)  [unwired: 4 in, 1 out]
            n80 = call <vilib>:"Add State(s) to Queue__jki_lib_state_machine.vi"("State(s) in (\"\")"=w228) -> ("States Out"=w227:string)  [unwired: 14 in]
          }
          frame "UI: Cursor Set" {
            # "Argument"
            # "Initialize the User Interface, here.\n(this is called automatically, by the Macro: Init)"
            n81 = disable-structure shown="Default" {
              disable-tunnel: w231 -> [w236 w239]
              disable-tunnel: [w236 w238] -> w230
              disable-tunnel: w229 -> [_ w237]
              frame condition #0 {
              }
              frame condition #1 (active) {
                n82 = case shown="\"Idle\", Default" w237 {
                  tunnel: w239 -> [w241 w243]
                  tunnel: [w240 w242] -> w238
                  frame "Idle", Default {
                    n83 = call <vilib>:"Unset Busy.vi"("error in (no error)"=w241) -> ("error out"=w240:errorcluster)  [unwired: 10 in]
                  }
                  frame "Busy" {
                    n84 = call <vilib>:"Set Busy.vi"("error in (no error)"=w243) -> ("error out"=w242:errorcluster)  [unwired: 9 in, 1 out]
                  }
                }
              }
            }
            n85 = call <vilib>:"Add State(s) to Queue__jki_lib_state_machine.vi"("State(s) in (\"\")"=w235) -> ("States Out"=w234:string)  [unwired: 14 in]
          }
          frame "UI: Front Panel State" {
            # "Argument"
            # "Set Front Panel Open or Closed\n(Usage: \"UI: Front Panel State >> Open|Close\")"
            n86 = Unbundle By Name(w247) -> ("Core.Current VI Reference"=w246:refnum<vi>)
            n87 = disable-structure shown="Default" {
              disable-tunnel: w249 -> [w255 w278]
              disable-tunnel: [w254 w278] -> w248
              disable-tunnel: w246 -> [w253 _]
              disable-tunnel: w245 -> [w252 _]
              frame condition #0 (active) {
                n88 = case shown="\"Close\"" w252 {
                  tunnel: w255 -> [w259 w272]
                  tunnel: [w261 w273] -> w254
                  tunnel: w253 -> [w260 w270]
                  frame "Open", Default {
                    n89 = property class="VI"(reference=w260, error in=w259) -> (reference out=w257:refnum<vi>, error out=w258:errorcluster, "FP.State"=w256:T8)
                    n90 = case shown="\"Closed\"" w256 {
                      tunnel: [w264 w267] -> w261
                      tunnel: w258 -> [w263 w267]
                      tunnel: w257 -> [w262 _]
                      frame "Closed" {
                        n91 = invoke class="VI" method="FP.Open"(reference=w262, error in=w263, "Activate"=TRUE, "State"=T8."Standard") -> (error out=w264:errorcluster)  [unwired: 1 in, 4 out]
                      }
                      frame Default {
                      }
                    }
                  }
                  frame "Close" {
                    n92 = property class="VI"(reference=w270, error in=w272) -> (reference out=w269:refnum<vi>, error out=w271:errorcluster, "FP.State"=w268:T8)
                    n93 = case shown="Default" w268 {
                      tunnel: [w274 w277] -> w273
                      tunnel: w271 -> [w274 w276]
                      tunnel: w269 -> [_ w275]
                      frame "Invalid", "Closed" {
                      }
                      frame Default {
                        n94 = invoke class="VI" method="FP.Close"(reference=w275, error in=w276) -> (error out=w277:errorcluster)  [unwired: 1 in, 2 out]
                      }
                    }
                  }
                }
              }
              frame condition #1 {
              }
            }
            n95 = call <vilib>:"Add State(s) to Queue__jki_lib_state_machine.vi"("State(s) in (\"\")"=w251) -> ("States Out"=w250:string)  [unwired: 14 in]
          }
          frame "---------- Macro ----------" {
            # "Do not put any code in this frame.\n(It is a separator no-op. You can make a copy of this frame to create a new Macro frame)"
            n96 = call <vilib>:"Add State(s) to Queue__jki_lib_state_machine.vi"("State(s) in (\"\")"=w283) -> ("States Out"=w282:string)  [unwired: 14 in]
          }
          frame "Macro: Initialize" {
            w285 = "UI: Initialize\nUI: Front Panel State >> Close\nMacro: Debug\nInstrument: Open\nInstrument: getAll"  # UI: Initialize UI: Front Panel State >> Close Macro: Debug Instrument: Open Instrument: getAll
            # "Initialization Macro\n(This is called once, when the VI starts)"
            n97 = call <vilib>:"Add State(s) to Queue__jki_lib_state_machine.vi"("State(s) in Front (\"\")"="Data: Initialize\nInitialize Core Data\nEvents: Register", "State(s) in (\"\")"="Process: Sync", "State(s) at Back (\"\")"=w285) -> ("States Out"=w287:string)  [unwired: 12 in]
            n98 = call <vilib>:"Add State(s) to Queue__jki_lib_state_machine.vi"("State(s) in Front (\"\")"=w287, "State(s) in (\"\")"=w292) -> ("States Out"=w291:string)  [unwired: 13 in]
          }
          frame "Macro: Exit" {
            # "Exit Macro\n(This is called once, when the VI exits)"
            n99 = Unbundle By Name(w293) -> ("Core.Close Panel on Exit?"=w306:bool)
            n100 = Bundle By Name(cluster=w293, "Core.Shutdown?"=TRUE) -> (w294:T12)
            n101 = Select(t="UI: Front Panel State >> Close", s=w306, f="") -> (s? t:f=w303:string)
            n102 = call <vilib>:"Add State(s) to Queue__jki_lib_state_machine.vi"("State(s) in Front (\"\")"="Data: Cleanup\nEvents: Unregister", "State(s) in (\"\")"="Process: Sync", "State(s) at Back (\"\")"="Exit") -> ("States Out"=w298:string)  [unwired: 12 in]
            n103 = call <vilib>:"Add State(s) to Queue__jki_lib_state_machine.vi"("State(s) in Front (\"\")"="Instrument: Close", "State(s) in (\"\")"=w303, "State(s) at Back (\"\")"=w298) -> ("States Out"=w302:string)  [unwired: 12 in]
            n104 = call <vilib>:"Add State(s) to Queue__jki_lib_state_machine.vi"("State(s) in Front (\"\")"=w302, "State(s) in (\"\")"=w309) -> ("States Out"=w308:string)  [unwired: 13 in]
          }
          frame "Macro: Debug" {
            # "exe?"
            # "If pane is an EXE, then close it when we exit"
            # "Macro: Debug\n(get debug behavior, determine UI and determine shutdown behavior)"
            n105 = Unbundle By Name(w311) -> ("Core.Close Panel on Exit?"=w316:bool, "SMO"=w321:refnum<class "Instrument.Oxford1820.lvclass">)
            n106 = property class="App"() -> ("App.Kind"=w319:T5)  [unwired: 2 in, 2 out]
            n107 = Equal?(x=w319, y=T5."Run Time System" ("Application:Kind")) -> (x = y?=w315:bool)
            n108 = call <userlib>:"Get Debug Mode.vi"("error in (no error)"=w313, "SMO"=w321) -> ("error out"=w314:errorcluster, "Behavior"=w320:T14)  [unwired: 7 in, 1 out]
            n109 = case shown="\"Debug\"" w320 {
              tunnel: [w325 w327] -> w317
              tunnel: w316 -> [w325 _]
              tunnel: w315 -> [_ w329]
              tunnel: [_ w326] -> w310
              frame "Normal", Default {
                # "respect core.close"
              }
              frame "Debug" {
                w326 = "UI: Front Panel State >> Open\nSequence: Wait >> RESET\nSequence: Wait >> 1000"  # UI: Front Panel State >> Open Sequence: Wait >> RESET Sequence: Wait >> 1000
                # "keep panel open\nunless exe"
                n110 = Or(x=w329, y=FALSE) -> (x .or. y?=w327:bool)
              }
            }
            n111 = Bundle By Name(cluster=w311, "Core.Close Panel on Exit?"=w317) -> (w312:T12)
            n112 = call <vilib>:"Add State(s) to Queue__jki_lib_state_machine.vi"("State(s) in Front (\"\")"=w310, "State(s) in (\"\")"=w324) -> ("States Out"=w323:string)  [unwired: 13 in]
          }
          frame "Macro: Run Sequence" {
            # "0,1,2,3,4,"
            # "5"
            n113 = Unbundle By Name(w335) -> ("sequence"=w341:string[], "Running Step"=w333:i32)
            n114 = Index Array(array=w341, index=w333) -> (element=w339:string)
            n115 = Array Size(array=w341) -> (size(s)=w330:i32)
            n116 = Equal?(x=w330, y=w333) -> (x = y?=w334:bool)
            n117 = Select(t=-1 ("Running Step"), s=w334, f=w333) -> (s? t:f=w340:i32)
            n118 = Select(t="Data: Update Status >> ...", s=w334, f="Idle\nMacro: Run Sequence" ("State(s) at Back (\"\")")) -> (s? t:f=w336:string)
            n119 = Bundle By Name(cluster=w335, "Running Step"=w340) -> (w342:T12)
            n120 = call <vilib>:"Add State(s) to Queue__jki_lib_state_machine.vi"("State(s) in Front (\"\")"=w339, "State(s) at Back (\"\")"=w336) -> ("States Out"=w338:string)  [unwired: 13 in]
            n121 = call <vilib>:"Add State(s) to Queue__jki_lib_state_machine.vi"("State(s) in Front (\"\")"=w338, "State(s) in (\"\")"=w346) -> ("States Out"=w345:string)  [unwired: 13 in]
          }
          frame "Macro: Post Error Handling" {
            # "Clear Last Error?"
            n122 = Unbundle By Name(w350) -> ("Core.Last Error.remaining states"=w356:string, "Core.Shutdown?"=w357:bool)
            n123 = Unbundle By Name(w350) -> ("Core.Last Error.error"=w353:errorcluster)
            n124 = case shown="False" FALSE {
              tunnel: w353 -> [w359 _]
              tunnel: [w359 _] -> w352
              frame False {
              }
              frame True {
              }
            }
            n125 = case shown="True" w357 {
              tunnel: w356 -> [w360 w362]
              tunnel: [w360 w361] -> w355
              frame False {
                # "These are the remaining states (at the moment the error occured). States can be altered according to business logic."
                # "NOT SHUTTING DOWN"
              }
              frame True {
                # "Developer can decide to alter the states but should be aware that during the shutdown process, there are certain states that must be run for the SMO to properly shut itself (and this process) down. As such, one can add states to perform additional clean-ups, but should append the remaining state to be executed."
                # "SHUTTING DOWN"
                n126 = call <vilib>:"Add State(s) to Queue__jki_lib_state_machine.vi"("State(s) in (\"\")"=w362) -> ("States Out"=w361:string)  [unwired: 14 in]
              }
            }
            n127 = Bundle By Name(cluster=w350, "Core.Last Error.error"=w352) -> (w347:T12)
            n128 = call <vilib>:"Add State(s) to Queue__jki_lib_state_machine.vi"("State(s) in Front (\"\")"=w355, "State(s) in (\"\")"=w349) -> ("States Out"=w348:string)  [unwired: 13 in]
          }
          frame "Macro: Load SetMagnet Sequence" {
            # "clear the queue"
            # "LOAD.\n(It is a separator no-op. You can make a copy of this frame to create a new Macro frame)"
            n129 = Unbundle By Name(w366) -> ("setMagnet.mode"=w381:T3)
            n130 = Unbundle By Name(w366) -> ("SMO"=w365:refnum<class "Instrument.Oxford1820.lvclass">, "setMagnet.field"=w373:dbl)
            n131 = Equal?(x=Magnet_Mode--Enum."Persistent", y=w381) -> (x = y?=w371:bool)
            n132 = Unbundle By Name(w365) -> ("1820_IPS_Magnet_Field"=w364:dbl)
            n133 = Select(t="Sequence: Switch >> Off\nSequence: Wait >> RESET\nSequence: Wait >> 30000\nSequence: Ramp PSU to Zero\nSequence: Check Hold" ("State(s) in Front (\"\")"), s=w371, f="") -> (s? t:f=w369:string)
            n134 = call <vilib>:"Add State(s) to Queue__jki_lib_state_machine.vi"("State(s) in Front (\"\")"="Sequence: Hold\nSequence: Check Hold\nSequence: Ramp PSU to Magnet\nSequence: Check Hold\nSequence: Switch >> On\nSequence: Wait >> RESET\nSequence: Wait >> 30000\nSequence: Ramp PSU to Target\nSequence: Check Hold" ("State(s) in Front (\"\")"), "State(s) in (\"\")"=w369, "State(s) at Back (\"\")"="") -> ("States Out"=w372:string)  [unwired: 12 in]
            n135 = call "Instrument.1820.FloatApprox.vi"("y"=w373, "x"=w364) -> ("x ~ y?"=w374:bool)  [unwired: 4 in]
            n136 = call <userlib>:"String to 1D Array__ogtk.vi"("delimiter (Tab)"="\n", "string"=w372) -> ("Array of Strings"=w378:string[])  [unwired: 9 in]
            n137 = case shown="False" w374 {
              tunnel: w378 -> [w387 _]
              tunnel: ["Macro: Run Sequence" ("State(s) in Front (\"\")") "" ("State(s) in Front (\"\")")] -> w377
              tunnel: [w385 w389] -> w375
              tunnel: w366 -> [w384 w389]
              frame False {
                n138 = Bundle By Name(cluster=w384, "Running Step"=0 ("sequence"), "sequence"=w387) -> (w385:T12)
              }
              frame True {
              }
            }
            n139 = call <vilib>:"Add State(s) to Queue__jki_lib_state_machine.vi"("State(s) in Front (\"\")"=w377) -> ("States Out"=w383:string)  [unwired: 14 in]
          }
          frame "Macro: Abort SetMagnet Sequence" {
            # "clear the queue"
            # "ABORT\n(It is a separator no-op. You can make a copy of this frame to create a new Macro frame)"
            n140 = call <userlib>:"String to 1D Array__ogtk.vi"("delimiter (Tab)"="\n", "string"="" ("State(s) in Front (\"\")")) -> ("Array of Strings"=w398:string[])  [unwired: 9 in]
            n141 = Bundle By Name(cluster=w393, "Running Step"=0 ("sequence"), "sequence"=w398) -> (w395:T12)
            n142 = call <vilib>:"Add State(s) to Queue__jki_lib_state_machine.vi"("State(s) in Front (\"\")"="Macro: Run Sequence" ("State(s) in Front (\"\")")) -> ("States Out"=w400:string)  [unwired: 14 in]
          }
          frame "---------- Process ----------" {
            # "Template Separator\n(You can make a copy of, or modify, this frame)"
            n143 = call <vilib>:"Add State(s) to Queue__jki_lib_state_machine.vi"("State(s) in (\"\")"=w405) -> ("States Out"=w404:string)  [unwired: 14 in]
          }
          frame "Process: Sync" {
            n144 = Unbundle By Name(w413) -> ("SMO"=w409:refnum<class "Instrument.Oxford1820.lvclass">)
            n145 = call <vilib>:"WaitOnProcessSync.vi"("error in (no error)"=w408, "SMO"=w409) -> ("error out"=w407:errorcluster, "Don't run?"=w412:bool)  [unwired: 7 in, 1 out]
            n146 = Select(t="Data: Cleanup\nEvents: Unregister\nExit", s=w412, f="") -> (s? t:f=w406:string)
            n147 = call <vilib>:"Add State(s) to Queue__jki_lib_state_machine.vi"("State(s) in Front (\"\")"=w406, "State(s) in (\"\")"=w416) -> ("States Out"=w415:string)  [unwired: 13 in]
          }
          frame "---------- Events ----------" {
            # "Template Separator\n(You can make a copy of, or modify, this frame)"
            n148 = call <vilib>:"Add State(s) to Queue__jki_lib_state_machine.vi"("State(s) in (\"\")"=w421) -> ("States Out"=w420:string)  [unwired: 14 in]
          }
          frame "Events: Register" {
            # "Expand to add\nmore events"
            n149 = Unbundle By Name(w432) -> ("SMO"=w429:refnum<class "Instrument.Oxford1820.lvclass">)
            n150 = call <vilib>:"GetProtectedEvents.vi"("SMO"=w429) -> ("error out"=w425:errorcluster, "SMO Protected Events"=w430:T15, "SMO out"=w424:refnum<class "Instrument.Oxford1820.lvclass">)  [unwired: 8 in]
            n151 = call "Instrument.Oxford1820.GetPrivateEvents.vi"("Instrument.Oxford1820"=w424) -> ("error out"=w423:errorcluster, "Instrument.Oxford1820.Private Events"=w422:T16)  [unwired: 8 in, 1 out]
            n152 = register-events(w430, w422) -> (reference out=w431:refnum<event-registration>, error out=w426:errorcluster)  [unwired: 2 in]
            n153 = Merge Errors(w423, w428, w426, w425) -> (w427:errorcluster)
            n154 = call <vilib>:"Add State(s) to Queue__jki_lib_state_machine.vi"("State(s) in (\"\")"=w434) -> ("States Out"=w433:string)  [unwired: 14 in]
          }
          frame "Events: Unregister" {
            n155 = Unregister For Events(event registration refnum=w437, error in=w436) -> (error out=w435:errorcluster)
            n156 = call <vilib>:"Clear Errors.vi"("error in (no error)"=w435) -> ()  [unwired: 5 in, 2 out]
            n157 = call <vilib>:"Add State(s) to Queue__jki_lib_state_machine.vi"("State(s) in (\"\")"=w440) -> ("States Out"=w439:string)  [unwired: 14 in]
          }
          frame "---------- Instrument ----------" {
            n158 = Unbundle By Name(w442) -> ("SMO"=w443:refnum<class "Instrument.Oxford1820.lvclass">)
            n159 = Bundle By Name(cluster=w442, "SMO"=w443) -> (w441:T12)
            n160 = call <vilib>:"Add State(s) to Queue__jki_lib_state_machine.vi"("State(s) in (\"\")"=w447) -> ("States Out"=w446:string)  [unwired: 14 in]
          }
          frame "Instrument: Open" {
            n161 = Unbundle By Name(w452) -> ("SMO"=w453:refnum<class "Instrument.Oxford1820.lvclass">)
            n162 = call-dynamic "Open Hardware.vi"("error in (no error)"=w449, "Instrument.Oxford1820 in"=w453) -> ("error out"=w448:errorcluster, "Instrument.Oxford1820 out"=w451:refnum<class "Instrument.Oxford1820.lvclass">)  [unwired: 8 in]
            n163 = Bundle By Name(cluster=w452, "SMO"=w451) -> (w450:T12)
            n164 = call <vilib>:"Add State(s) to Queue__jki_lib_state_machine.vi"("State(s) in (\"\")"=w456) -> ("States Out"=w455:string)  [unwired: 14 in]
          }
          frame "Instrument: Close" {
            n165 = Unbundle By Name(w461) -> ("SMO"=w462:refnum<class "Instrument.Oxford1820.lvclass">)
            n166 = call-dynamic "Close Hardware.vi"("error in (no error)"=w458, "Instrument.Oxford1820 in"=w462) -> ("error out"=w457:errorcluster, "Instrument.Oxford1820 out"=w460:refnum<class "Instrument.Oxford1820.lvclass">)  [unwired: 8 in]
            n167 = Bundle By Name(cluster=w461, "SMO"=w460) -> (w459:T12)
            n168 = call <vilib>:"Add State(s) to Queue__jki_lib_state_machine.vi"("State(s) in (\"\")"=w465) -> ("States Out"=w464:string)  [unwired: 14 in]
          }
          frame "Instrument: getAll" {
            n169 = Unbundle By Name(w474) -> ("SMO"=w471:refnum<class "Instrument.Oxford1820.lvclass">)
            n170 = call "Instrument.Oxford1820.getAll.vi"("error in (no error)"=w472, "Instrument.Oxford1820 in"=w471) -> ("error out"=w468:errorcluster, "output cluster"=w466:T17, "Instrument.Oxford1820 out"=w470:refnum<class "Instrument.Oxford1820.lvclass">)  [unwired: 7 in]
            n171 = call <userlib>:"setAllData.vi"("error in (no error)"=w468, "AllData"=w466, "Instrument in"=w470) -> ("error out"=w467:errorcluster, "Instrument out"=w469:refnum<class "Instrument.Oxford1820.lvclass">)  [unwired: 7 in]
            n172 = Bundle By Name(cluster=w474, "SMO"=w469) -> (w473:T12)
            n173 = call <vilib>:"Add State(s) to Queue__jki_lib_state_machine.vi"("State(s) in (\"\")"=w477) -> ("States Out"=w476:string)  [unwired: 14 in]
          }
          frame "Instrument: Log" {
            n174 = Unbundle By Name(w487) -> ("SMO"=w482:refnum<class "Instrument.Oxford1820.lvclass">)
            n175 = Unbundle By Name(w482) -> ("getAll"=w481:T17)
            n176 = call-dynamic "Get SMO Database Paths.vi"("error in (no error)"=w479, "Instrument.Oxford1820 in"=w482) -> ("error out"=w480:errorcluster, "Paths"=w483:string, "Instrument.Oxford1820 out"=w484:refnum<class "Instrument.Oxford1820.lvclass">)  [unwired: 7 in]
            n177 = call <userlib>:"Instrument.logToDatabase.vi"("error in (no error)"=w480, "Data"=w481, "Paths"=w483, "Instrument"=w484) -> ("error out"=w478:errorcluster, "Instrument out"=w485:refnum<class "Instrument.Oxford1820.lvclass">)  [unwired: 6 in]
            n178 = Bundle By Name(cluster=w487, "SMO"=w485) -> (w486:T12)
            n179 = call <vilib>:"Add State(s) to Queue__jki_lib_state_machine.vi"("State(s) in (\"\")"=w490) -> ("States Out"=w489:string)  [unwired: 14 in]
          }
          frame "Instrument: setAction" {
            # "#todo\n- Add a state for each action (Instrument: Hold) instead of Instrument: setAction >> Hold\n- Use data wire (ie Message.Data or Target cluster) to pass data instead of using arguments"
            # "allow easy way for\nlocal states to call this state"
            n180 = Unbundle By Name(w496) -> ("SMO"=w499:refnum<class "Instrument.Oxford1820.lvclass">, "Message.Data"=w495:variant)
            n181 = case shown="\"\"" w493 {
              selector: w493 -> [w505 _]
              tunnel: [w505 w509] -> w498
              tunnel: [w504 w508] -> w497
              tunnel: w495 -> [_ w507]
              tunnel: w494 -> [w504 w506]
              frame Default {
              }
              frame "" {
                n182 = call "JSON to LVtype.vim"("type"=T9 "HOLD" ("PSU Act Stat"), "error in (no error)"=w506, "JSON Data in"=w507) -> ("error out"=w508:errorcluster, "Data out"=w509:T9)  [unwired: 7 in]
              }
            }
            n183 = call "Set IPS Action.vi"("error in (no error)"=w497, "PSU Act Stat"=w498, "Instrument.Oxford1820 in"=w499) -> ("error out"=w491:errorcluster, "Instrument.Oxford1820 out"=w492:refnum<class "Instrument.Oxford1820.lvclass">)  [unwired: 6 in, 1 out]
            n184 = Bundle By Name(cluster=w496, "SMO"=w492) -> (w500:T12)
            n185 = call <vilib>:"Add State(s) to Queue__jki_lib_state_machine.vi"("State(s) in (\"\")"=w503) -> ("States Out"=w502:string)  [unwired: 14 in]
          }
          frame "Instrument: Hold" {
            n186 = Unbundle By Name(w515) -> ("SMO"=w516:refnum<class "Instrument.Oxford1820.lvclass">)  [unwired: 1 out]
            n187 = call "Set IPS Action.vi"("error in (no error)"=w513, "PSU Act Stat"=T9 "HOLD", "Instrument.Oxford1820 in"=w516) -> ("error out"=w511:errorcluster, "Instrument.Oxford1820 out"=w512:refnum<class "Instrument.Oxford1820.lvclass">)  [unwired: 6 in, 1 out]
            n188 = Bundle By Name(cluster=w515, "SMO"=w512) -> (w517:T12)
            n189 = call <vilib>:"Add State(s) to Queue__jki_lib_state_machine.vi"("State(s) in (\"\")"=w520) -> ("States Out"=w519:string)  [unwired: 14 in]
          }
          frame "Instrument: Clamp" {
            n190 = Unbundle By Name(w526) -> ("SMO"=w529:refnum<class "Instrument.Oxford1820.lvclass">)  [unwired: 1 out]
            n191 = Two Button Dialog(message="Clamp output:\nAre you sure?", 1:"No" ("F button name (\"Cancel\")"), 2:"Yes" ("T button name (\"OK\")")) -> (T button?=w521:bool)
            n192 = case shown="True" w521 {
              tunnel: w529 -> [w535 w540]
              tunnel: [w535 w537] -> w528
              tunnel: [w534 w536] -> w527
              tunnel: w525 -> [w534 w538]
              frame False {
              }
              frame True {
                n193 = call "Set IPS Action.vi"("error in (no error)"=w538, "PSU Act Stat"=T9 "CLMP", "Instrument.Oxford1820 in"=w540) -> ("error out"=w536:errorcluster, "Instrument.Oxford1820 out"=w537:refnum<class "Instrument.Oxford1820.lvclass">)  [unwired: 6 in, 1 out]
              }
            }
            n194 = Bundle By Name(cluster=w526, "SMO"=w528) -> (w530:T12)
            n195 = call <vilib>:"Add State(s) to Queue__jki_lib_state_machine.vi"("State(s) in (\"\")"=w533) -> ("States Out"=w532:string)  [unwired: 14 in]
          }
          frame "Instrument: RampToSet" {
            n196 = Unbundle By Name(w545) -> ("SMO"=w546:refnum<class "Instrument.Oxford1820.lvclass">)  [unwired: 1 out]
            n197 = call "Set IPS Action.vi"("error in (no error)"=w543, "PSU Act Stat"=T9 "RTOS", "Instrument.Oxford1820 in"=w546) -> ("error out"=w542:errorcluster, "Instrument.Oxford1820 out"=w541:refnum<class "Instrument.Oxford1820.lvclass">)  [unwired: 6 in, 1 out]
            n198 = Bundle By Name(cluster=w545, "SMO"=w541) -> (w547:T12)
            n199 = call <vilib>:"Add State(s) to Queue__jki_lib_state_machine.vi"("State(s) in (\"\")"=w550) -> ("States Out"=w549:string)  [unwired: 14 in]
          }
          frame "Instrument: RampToZero" {
            n200 = Unbundle By Name(w555) -> ("SMO"=w556:refnum<class "Instrument.Oxford1820.lvclass">)  [unwired: 1 out]
            n201 = call "Set IPS Action.vi"("error in (no error)"=w553, "PSU Act Stat"=T9 "RTOZ", "Instrument.Oxford1820 in"=w556) -> ("error out"=w551:errorcluster, "Instrument.Oxford1820 out"=w552:refnum<class "Instrument.Oxford1820.lvclass">)  [unwired: 6 in, 1 out]
            n202 = Bundle By Name(cluster=w555, "SMO"=w552) -> (w557:T12)
            n203 = call <vilib>:"Add State(s) to Queue__jki_lib_state_machine.vi"("State(s) in (\"\")"=w560) -> ("States Out"=w559:string)  [unwired: 14 in]
          }
          frame "Instrument: setTarget" {
            n204 = Unbundle By Name(w562) -> ("SMO"=w569:refnum<class "Instrument.Oxford1820.lvclass">)
            n205 = case shown="\"\"" w565 {
              selector: w565 -> [w579 _]
              tunnel: [w577 w580] -> w568
              tunnel: [w576 w583] -> w567
              tunnel: w566 -> [w574 w581]
              tunnel: [w575 w581] -> w561
              tunnel: w562 -> [_ w582]
              frame Default {
                n206 = Scan From String(format string="%f %f", input string=w579, error in=w574) -> (error out=w575:errorcluster, output 1=w577:dbl, output 2=w576:dbl)  [unwired: 3 in, 2 out]
              }
              frame "" {
                n207 = Unbundle By Name(w582) -> ("setMagnet.field"=w580:dbl, "setMagnet.rate"=w583:dbl)
              }
            }
            n208 = call "Set IPS PSU Targets.vi"("error in (no error)"=w561, "Target Field Rate (T/min)"=w567, "Target Field (T)"=w568, "Instrument.Oxford1820 in"=w569) -> ("error out"=w563:errorcluster, "Instrument.Oxford1820 out"=w564:refnum<class "Instrument.Oxford1820.lvclass">)  [unwired: 5 in, 1 out]
            n209 = Bundle By Name(cluster=w562, "SMO"=w564) -> (w570:T12)
            n210 = call <vilib>:"Add State(s) to Queue__jki_lib_state_machine.vi"("State(s) in (\"\")"=w573) -> ("States Out"=w572:string)  [unwired: 14 in]
          }
          frame "Instrument: setSwitchHeat" {
            # "this is a sequence!"
            n211 = Unbundle By Name(w594) -> ("SMO"=w590:refnum<class "Instrument.Oxford1820.lvclass">, "Message.Data"=w593:variant)
            n212 = case shown="\"\"" w584 {
              selector: w584 -> [w600 _]
              tunnel: w593 -> [_ w605]
              tunnel: [w600 w603] -> w591
              tunnel: [w599 w602] -> w587
              tunnel: w585 -> [w599 w601]
              frame Default {
              }
              frame "" {
                n213 = call "JSON to LVtype.vim"("type"=T10 "ON" ("Switch Heater Status"), "error in (no error)"=w601, "JSON Data in"=w605) -> ("error out"=w602:errorcluster, "Data out"=w603:T10)  [unwired: 7 in]
              }
            }
            n214 = call "Ramp PSU to Magnet.vi"("error in (no error)"=w587, "Instrument.Oxford1820 in"=w590) -> ("error out"=w586:errorcluster, "Instrument.Oxford1820 out"=w589:refnum<class "Instrument.Oxford1820.lvclass">)  [unwired: 8 in]
            n215 = call "Set IPS Switch Heater.vi"("error in (no error)"=w586, "Switch Heater Status"=w591, "Instrument.Oxford1820 in"=w589) -> ("error out"=w588:errorcluster, "Instrument.Oxford1820 out"=w592:refnum<class "Instrument.Oxford1820.lvclass">)  [unwired: 6 in, 1 out]
            n216 = Bundle By Name(cluster=w594, "SMO"=w592) -> (w595:T12)
            n217 = call <vilib>:"Add State(s) to Queue__jki_lib_state_machine.vi"("State(s) in (\"\")"=w598) -> ("States Out"=w597:string)  [unwired: 14 in]
          }
          frame "Instrument: setLambda" {
            n218 = Unbundle By Name(w614) -> ("SMO"=w611:refnum<class "Instrument.Oxford1820.lvclass">, "Message.Data"=w613:variant)
            n219 = call "JSON to LVtype.vim"("type"=T10 "ON" ("LPF State"), "error in (no error)"=w606, "JSON Data in"=w613) -> ("error out"=w609:errorcluster, "Data out"=w610:T10)  [unwired: 7 in]
            n220 = call "Set ITC LPF State.vi"("error in (no error)"=w609, "LPF State"=w610, "Instrument.Oxford1820 in"=w611) -> ("error out"=w608:errorcluster, "Instrument.Oxford1820 out"=w607:refnum<class "Instrument.Oxford1820.lvclass">)  [unwired: 6 in, 1 out]
            n221 = Bundle By Name(cluster=w614, "SMO"=w607) -> (w615:T12)
            n222 = call <vilib>:"Add State(s) to Queue__jki_lib_state_machine.vi"("State(s) in (\"\")"=w618) -> ("States Out"=w617:string)  [unwired: 14 in]
          }
          frame "Instrument: setFillMode" {
            n223 = Unbundle By Name(w627) -> ("SMO"=w625:refnum<class "Instrument.Oxford1820.lvclass">, "Message.Data"=w626:variant)
            n224 = call "JSON to LVtype.vim"("type"=T11 "ON" ("Fill Mode"), "error in (no error)"=w619, "JSON Data in"=w626) -> ("error out"=w623:errorcluster, "Data out"=w624:T11)  [unwired: 7 in]
            n225 = call "Set IPS Fill Mode.vi"("error in (no error)"=w623, "Fill Mode"=w624, "Instrument.Oxford1820 in"=w625) -> ("error out"=w622:errorcluster, "Instrument.Oxford1820 out"=w621:refnum<class "Instrument.Oxford1820.lvclass">)  [unwired: 6 in, 1 out]
            n226 = Bundle By Name(cluster=w627, "SMO"=w621) -> (w628:T12)
            n227 = call <vilib>:"Add State(s) to Queue__jki_lib_state_machine.vi"("State(s) in (\"\")"=w631) -> ("States Out"=w630:string)  [unwired: 14 in]
          }
          frame "Instrument: setNeedleValve" {
            n228 = Unbundle By Name(w640) -> ("SMO"=w635:refnum<class "Instrument.Oxford1820.lvclass">, "Message.Data"=w632:variant)
            n229 = call "JSON to LVtype.vim"("type"=0.0 ("Percentage Open (%)"), "error in (no error)"=w633, "JSON Data in"=w632) -> ("error out"=w638:errorcluster, "Data out"=w639:dbl)  [unwired: 7 in]
            n230 = call "Set ITC LPF Needle Valve.vi"("error in (no error)"=w638, "Percentage Open (%)"=w639, "Instrument.Oxford1820 in"=w635) -> ("error out"=w637:errorcluster, "Instrument.Oxford1820 out"=w636:refnum<class "Instrument.Oxford1820.lvclass">)  [unwired: 6 in, 1 out]
            n231 = Bundle By Name(cluster=w640, "SMO"=w636) -> (w641:T12)
            n232 = call <vilib>:"Add State(s) to Queue__jki_lib_state_machine.vi"("State(s) in (\"\")"=w644) -> ("States Out"=w643:string)  [unwired: 14 in]
          }
          frame "Instrument: getStatus" {
            n233 = Unbundle By Name(w649) -> ("SMO"=w645:refnum<class "Instrument.Oxford1820.lvclass">)
            n234 = call "Read IPS Status.vi"("error in (no error)"=w646, "Instrument.Oxford1820 in"=w645) -> ("error out"=w647:errorcluster, "Instrument.Oxford1820 out"=w648:refnum<class "Instrument.Oxford1820.lvclass">)  [unwired: 7 in, 1 out]
            n235 = Bundle By Name(cluster=w649, "SMO"=w648) -> (w650:T12)
            n236 = call <vilib>:"Add State(s) to Queue__jki_lib_state_machine.vi"("State(s) in (\"\")"=w653) -> ("States Out"=w652:string)  [unwired: 14 in]
          }
          frame "---------- Sequence ----------" {
            # "Do Not call these states directly: only call from a sequence array"
            n237 = Unbundle By Name(w656) -> ("Running Step"=w654:i32, "SMO"=w658:refnum<class "Instrument.Oxford1820.lvclass">)
            n238 = Increment(x=w654) -> (x+1=w657:i32)
            n239 = Bundle By Name(cluster=w656, "Running Step"=w657, "SMO"=w658) -> (w655:T12)
            n240 = call <vilib>:"Add State(s) to Queue__jki_lib_state_machine.vi"("State(s) in (\"\")"=w662) -> ("States Out"=w661:string)  [unwired: 14 in]
          }
          frame "Sequence: Wait" {
            # "F = repeat this state. wait\nT = go to next state. don't wait"
            n241 = Unbundle By Name(w671) -> ("Running Step"=w681:i32)
            n242 = call <userlib>:"Wait Logic.vi"("error in (no error)"=w669, "Time"=w668) -> ("error out"=w666:errorcluster, "Status String"=w663:string, "timer value"=→"timer":u32, "Trigger"=w667:bool)  [unwired: 6 in]
            n243 = Increment(x=w681) -> (x+1=w680:i32)
            n244 = Select(t=w680, s=w667, f=w681) -> (s? t:f=w679:i32)
            n245 = Select(t=u32 0, s=w667, f=u32 100 ("milliseconds to wait")) -> (s? t:f=w674:u32)
            n246 = Bundle By Name(cluster=w671, "Running Step"=w679) -> (w665:T12)
            n247 = call <userlib>:"Wait (ms)__ogtk.vi"("error in (no error)"=w666, "milliseconds to wait"=w674) -> ("error out"=w672:errorcluster)  [unwired: 8 in, 1 out]
            n248 = Format Into String(format string="%s", w663) -> (resulting string=w676:string)  [unwired: 2 in, 1 out]
            n249 = call <vilib>:"Build State String with Arguments__JKI_lib_State_Machine.vi"("Arguments (\"\")"=w676, "State"="Data: Update Status") -> ("State with Arguments"=w670:string)  [unwired: 4 in]
            n250 = call <vilib>:"Add State(s) to Queue__jki_lib_state_machine.vi"("State(s) in Front (\"\")"=w670, "State(s) in (\"\")"=w684) -> ("States Out"=w683:string)  [unwired: 13 in]
          }
          frame "Sequence: Hold" {
            n251 = Unbundle By Name(w693) -> ("Running Step"=w691:i32)
            n252 = Increment(x=w691) -> (x+1=w690:i32)
            n253 = Bundle By Name(cluster=w693, "Running Step"=w690) -> (w692:T12)
            n254 = Format Into String(format string="Instrument: setAction >> %s\nData: Update Status >> %s", T9 "HOLD" ("PSU Act Stat"), w687) -> (resulting string=w686:string)  [unwired: 2 in, 1 out]
            n255 = call <vilib>:"Add State(s) to Queue__jki_lib_state_machine.vi"("State(s) in Front (\"\")"=w686, "State(s) in (\"\")"=w696) -> ("States Out"=w695:string)  [unwired: 13 in]
          }
          frame "Sequence: Switch" {
            # "#todo: add abort public method"
            # "#todo: make these separate states\n1. check B = Target?\n2. Turn on switch\n3. set PSU to target\n4. check hold OR psu = target\n5. set persist mode"
            n256 = Unbundle By Name(w714) -> ("Running Step"=w706:i32, "SMO"=w700:refnum<class "Instrument.Oxford1820.lvclass">)
            n257 = case shown="\"Off\", Default" w710 {
              tunnel: [T10 "OFF" ("Switch Heater") T10 "ON" ("Switch Heater")] -> w704
              frame "Off", Default {
              }
              frame "On" {
              }
            }
            n258 = call "Read IPS Switch Heater.vi"("error in (no error)"=w697, "Instrument.Oxford1820 in"=w700) -> ("error out"=w698:errorcluster, "Switch Heater Status"=w699:string)  [unwired: 6 in, 2 out]
            n259 = Equal?(x=w699, y=w704) -> (x = y?=w707:bool)
            n260 = case shown="False" w707 {
              tunnel: w706 -> [w722 w727]
              tunnel: [w721 w724] -> w705
              tunnel: w704 -> [w719 _]
              tunnel: [w718 ""] -> w701
              frame False {
                # "+1 go to wait reset"
                n261 = Increment(x=w722) -> (x+1=w721:i32)
                n262 = Format Into String(format string="Instrument: setSwitchHeat >> %s", w719) -> (resulting string=w718:string)  [unwired: 2 in, 1 out]
              }
              frame True {
                # "if don't change switch,\nskip wait (+3)"
                n263 = Increment(x=w727) -> (x+1=w726:i32)
                n264 = Increment(x=w726) -> (x+1=w725:i32)
                n265 = Increment(x=w725) -> (x+1=w724:i32)
              }
            }
            n266 = Format Into String(format string="%s >> %s", w711, w710) -> (resulting string=w708:string)  [unwired: 2 in, 1 out]
            n267 = Bundle By Name(cluster=w714, "Running Step"=w705) -> (w713:T12)
            n268 = call <vilib>:"Build State String with Arguments__JKI_lib_State_Machine.vi"("Arguments (\"\")"=w708, "State"="Data: Update Status") -> ("State with Arguments"=w703:string)  [unwired: 4 in]
            n269 = call <vilib>:"Add State(s) to Queue__jki_lib_state_machine.vi"("State(s) in Front (\"\")"=w701, "State(s) at Back (\"\")"=w703) -> ("States Out"=w702:string)  [unwired: 13 in]
            n270 = call <vilib>:"Add State(s) to Queue__jki_lib_state_machine.vi"("State(s) in Front (\"\")"=w702, "State(s) in (\"\")"=w717) -> ("States Out"=w716:string)  [unwired: 13 in]
          }
          frame "Sequence: Ramp PSU to Target" {
            # "#todo: this whole frame is a sequence!"
            # "#todo: add abort public method"
            # "#todo: make these separate states\n1. check B = Target?\n2. Turn on switch\n3. set PSU to target\n4. check hold OR psu = target\n5. set persist mode"
            n271 = Unbundle By Name(w746) -> ("Running Step"=w732:i32, "sequence"=w731:string[], "SMO"=w737:refnum<class "Instrument.Oxford1820.lvclass">, "setMagnet.field"=w739:dbl, "setMagnet.rate"=w738:dbl)
            n272 = call "Read IPS PSU Field.vi"("error in (no error)"=w734, "Instrument.Oxford1820 in"=w737) -> ("error out"=w735:errorcluster, "Power Supply Field (T)"=w736:dbl)  [unwired: 7 in, 1 out]
            n273 = Increment(x=w732) -> (x+1=w730:i32)
            n274 = call "Instrument.1820.FloatApprox.vi"("y"=w739, "x"=w736) -> ("x ~ y?"=w747:bool)  [unwired: 4 in]
            n275 = case shown="False" w747 {
              tunnel: [w757 ""] -> w742
              tunnel: w739 -> [w755 _]
              tunnel: w738 -> [w754 _]
              tunnel: w731 -> [w751 w758]
              tunnel: [w751 w758] -> w733
              tunnel: w730 -> [w752 _]
              frame False {
                n276 = Format Into String(format string="Instrument: setTarget >> %f %f\nInstrument: RampToSet" ("State"), w755, w754) -> (resulting string=w757:string)  [unwired: 2 in, 1 out]
                n277 = Insert Into Array(array=w751, index=w752, new element="Sequence: Check RTOS" ("State")) -> ()  [unwired: 1 out]
              }
              frame True {
                # "If PSU Field == Target, do nothing"
              }
            }
            n278 = call <vilib>:"Build State String with Arguments__JKI_lib_State_Machine.vi"("Arguments (\"\")"=w744, "State"="Data: Update Status") -> ("State with Arguments"=w740:string)  [unwired: 4 in]
            n279 = Bundle By Name(cluster=w746, "Running Step"=w730, "sequence"=w733) -> (w745:T12)
            n280 = call <vilib>:"Add State(s) to Queue__jki_lib_state_machine.vi"("State(s) in Front (\"\")"=w742, "State(s) at Back (\"\")"=w740) -> ("States Out"=w741:string)  [unwired: 13 in]
            n281 = call <vilib>:"Add State(s) to Queue__jki_lib_state_machine.vi"("State(s) in Front (\"\")"=w741, "State(s) in (\"\")"=w750) -> ("States Out"=w749:string)  [unwired: 13 in]
          }
          frame "Sequence: Ramp PSU to Magnet" {
            # "#todo: add abort public method"
            # "#todo: make these separate states\n1. check B = Target?\n2. Turn on switch\n3. set PSU to target\n4. check hold OR psu = target\n5. set persist mode"
            n282 = Unbundle By Name(w779) -> ("Running Step"=w777:i32, "sequence"=w765:string[], "SMO"=w772:refnum<class "Instrument.Oxford1820.lvclass">)
            n283 = call "Read IPS PSU Field.vi"("error in (no error)"=w768, "Instrument.Oxford1820 in"=w772) -> ("error out"=w770:errorcluster, "Power Supply Field (T)"=w773:dbl, "Instrument.Oxford1820 out"=w771:refnum<class "Instrument.Oxford1820.lvclass">)  [unwired: 7 in]
            n284 = call "Read IPS Magnet Field.vi"("error in (no error)"=w770, "Instrument.Oxford1820 in"=w771) -> ("error out"=w769:errorcluster, "Magnet Field (T)"=w761:dbl)  [unwired: 7 in, 1 out]
            n285 = Increment(x=w777) -> (x+1=w764:i32)
            n286 = call "Instrument.1820.FloatApprox.vi"("y"=w761, "x"=w773) -> ("x ~ y?"=w767:bool)  [unwired: 4 in]
            n287 = case shown="False" w767 {
              tunnel: [w789 ""] -> w762
              tunnel: w761 -> [w787 _]
              tunnel: 1.0 -> [w786 _]
              tunnel: w765 -> [w783 w790]
              tunnel: [w783 w790] -> w763
              tunnel: w764 -> [w784 _]
              frame False {
                n288 = Format Into String(format string="Instrument: setTarget >> %f %f\nInstrument: RampToSet" ("State"), w787, w786) -> (resulting string=w789:string)  [unwired: 2 in, 1 out]
                n289 = Insert Into Array(array=w783, index=w784, new element="Sequence: Check RTOS" ("State")) -> ()  [unwired: 1 out]
              }
              frame True {
                # "If PSU Field == Target, do nothing"
              }
            }
            n290 = call <vilib>:"Build State String with Arguments__JKI_lib_State_Machine.vi"("Arguments (\"\")"=w776, "State"="Data: Update Status") -> ("State with Arguments"=w775:string)  [unwired: 4 in]
            n291 = Bundle By Name(cluster=w779, "Running Step"=w764, "sequence"=w763) -> (w778:T12)
            n292 = call <vilib>:"Add State(s) to Queue__jki_lib_state_machine.vi"("State(s) in Front (\"\")"=w762, "State(s) at Back (\"\")"=w775) -> ("States Out"=w774:string)  [unwired: 13 in]
            n293 = call <vilib>:"Add State(s) to Queue__jki_lib_state_machine.vi"("State(s) in Front (\"\")"=w774, "State(s) in (\"\")"=w782) -> ("States Out"=w781:string)  [unwired: 13 in]
          }
          frame "Sequence: Ramp PSU to Zero" {
            # "#todo: add abort public method"
            # "#todo: make these separate states\n1. check B = Target?\n2. Turn on switch\n3. set PSU to target\n4. check hold OR psu = target\n5. set persist mode"
            n294 = Unbundle By Name(w801) -> ("Running Step"=w799:i32, "sequence"=w792:string[])
            n295 = Increment(x=w799) -> (x+1=w793:i32)
            n296 = Format Into String(format string="Instrument: RampToZero\nData: Update Status >> %s", w797) -> (resulting string=w796:string)  [unwired: 2 in, 1 out]
            n297 = Insert Into Array(array=w792, index=w793, new element="Sequence: Check RTOZ" ("State")) -> ()  [unwired: 1 out]
            n298 = Bundle By Name(cluster=w801, "Running Step"=w793, "sequence"=w792) -> (w800:T12)
            n299 = call <vilib>:"Add State(s) to Queue__jki_lib_state_machine.vi"("State(s) in Front (\"\")"=w796, "State(s) in (\"\")"=w804) -> ("States Out"=w803:string)  [unwired: 13 in]
          }
          frame "Sequence: Check Hold" {
            # "F = repeat this state. wait\nT = go to next state. don't wait"
            n300 = Unbundle By Name(w819) -> ("Running Step"=w821:i32, "SMO"=w808:refnum<class "Instrument.Oxford1820.lvclass">)
            n301 = call "Read IPS Status.vi"("error in (no error)"=w805, "Instrument.Oxford1820 in"=w808) -> ("error out"=w806:errorcluster, "Status"=w807:string)  [unwired: 7 in, 1 out]
            n302 = call "Status String to Cluster.vi"("Status String"=w807) -> ("Status"=w810:T18)  [unwired: 10 in]
            n303 = Unbundle By Name(w810) -> ("Holding"=w812:bool)
            n304 = Increment(x=w821) -> (x+1=w822:i32)
            n305 = Select(t=w822, s=w812, f=w821) -> (s? t:f=w820:i32)
            n306 = Select(t=u32 0, s=w812, f=u32 500 ("milliseconds to wait")) -> (s? t:f=w814:u32)
            n307 = Bundle By Name(cluster=w819, "Running Step"=w820) -> (w818:T12)
            n308 = call <userlib>:"Wait (ms)__ogtk.vi"("error in (no error)"=w806, "milliseconds to wait"=w814) -> ("error out"=w811:errorcluster)  [unwired: 8 in, 1 out]
            n309 = call <vilib>:"Build State String with Arguments__JKI_lib_State_Machine.vi"("Arguments (\"\")"=w817, "State"="Data: Update Status") -> ("State with Arguments"=w816:string)  [unwired: 4 in]
            n310 = call <vilib>:"Add State(s) to Queue__jki_lib_state_machine.vi"("State(s) in Front (\"\")"=w816, "State(s) in (\"\")"=w825) -> ("States Out"=w824:string)  [unwired: 13 in]
          }
          frame "Sequence: Check RTOS" {
            # "F = repeat this state. wait\nT = go to next state. don't wait"
            n311 = Unbundle By Name(w840) -> ("Running Step"=w842:i32, "SMO"=w829:refnum<class "Instrument.Oxford1820.lvclass">)
            n312 = call "Read IPS Status.vi"("error in (no error)"=w826, "Instrument.Oxford1820 in"=w829) -> ("error out"=w827:errorcluster, "Status"=w828:string)  [unwired: 7 in, 1 out]
            n313 = call "Status String to Cluster.vi"("Status String"=w828) -> ("Status"=w830:T18)  [unwired: 10 in]
            n314 = Unbundle By Name(w830) -> ("Ramp to Setpoint"=w832:bool)
            n315 = Increment(x=w842) -> (x+1=w843:i32)
            n316 = Select(t=w843, s=w832, f=w842) -> (s? t:f=w841:i32)
            n317 = Select(t=u32 0, s=w832, f=u32 500 ("milliseconds to wait")) -> (s? t:f=w834:u32)
            n318 = Bundle By Name(cluster=w840, "Running Step"=w841) -> (w839:T12)
            n319 = call <userlib>:"Wait (ms)__ogtk.vi"("error in (no error)"=w827, "milliseconds to wait"=w834) -> ("error out"=w831:errorcluster)  [unwired: 8 in, 1 out]
            n320 = call <vilib>:"Build State String with Arguments__JKI_lib_State_Machine.vi"("Arguments (\"\")"=w837, "State"="Data: Update Status") -> ("State with Arguments"=w836:string)  [unwired: 4 in]
            n321 = call <vilib>:"Add State(s) to Queue__jki_lib_state_machine.vi"("State(s) in Front (\"\")"=w836, "State(s) in (\"\")"=w846) -> ("States Out"=w845:string)  [unwired: 13 in]
          }
          frame "Sequence: Check RTOZ" {
            # "F = repeat this state. wait\nT = go to next state. don't wait"
            n322 = Unbundle By Name(w861) -> ("Running Step"=w863:i32, "SMO"=w849:refnum<class "Instrument.Oxford1820.lvclass">)
            n323 = call "Read IPS Status.vi"("error in (no error)"=w847, "Instrument.Oxford1820 in"=w849) -> ("error out"=w848:errorcluster, "Status"=w850:string)  [unwired: 7 in, 1 out]
            n324 = call "Status String to Cluster.vi"("Status String"=w850) -> ("Status"=w851:T18)  [unwired: 10 in]
            n325 = Unbundle By Name(w851) -> ("Ramp to Zero"=w853:bool)
            n326 = Increment(x=w863) -> (x+1=w864:i32)
            n327 = Select(t=w864, s=w853, f=w863) -> (s? t:f=w862:i32)
            n328 = Bundle By Name(cluster=w861, "Running Step"=w862) -> (w860:T12)
            n329 = Select(t=u32 0, s=w853, f=u32 500 ("milliseconds to wait")) -> (s? t:f=w855:u32)
            n330 = call <userlib>:"Wait (ms)__ogtk.vi"("error in (no error)"=w848, "milliseconds to wait"=w855) -> ("error out"=w852:errorcluster)  [unwired: 8 in, 1 out]
            n331 = call <vilib>:"Build State String with Arguments__JKI_lib_State_Machine.vi"("Arguments (\"\")"=w858, "State"="Data: Update Status") -> ("State with Arguments"=w857:string)  [unwired: 4 in]
            n332 = call <vilib>:"Add State(s) to Queue__jki_lib_state_machine.vi"("State(s) in Front (\"\")"=w857, "State(s) in (\"\")"=w867) -> ("States Out"=w866:string)  [unwired: 13 in]
          }
          frame "Sequence: Check PSU at Zero" {
            # "F = repeat this state. wait\nT = go to next state. don't wait"
            n333 = Unbundle By Name(w885) -> ("Running Step"=w881:i32, "SMO"=w870:refnum<class "Instrument.Oxford1820.lvclass">)
            n334 = call "Read IPS PSU Field.vi"("error in (no error)"=w868, "Instrument.Oxford1820 in"=w870) -> ("error out"=w869:errorcluster, "Power Supply Field (T)"=w871:dbl)  [unwired: 7 in, 1 out]
            n335 = call "Instrument.1820.FloatApprox.vi"("y"=0.0, "x"=w871) -> ("x ~ y?"=w873:bool)  [unwired: 4 in]
            n336 = Increment(x=w881) -> (x+1=w882:i32)
            n337 = Select(t=w882, s=w873, f=w881) -> (s? t:f=w880:i32)
            n338 = Bundle By Name(cluster=w885, "Running Step"=w880) -> (w884:T12)
            n339 = Select(t=u32 0, s=w873, f=u32 500 ("milliseconds to wait")) -> (s? t:f=w875:u32)
            n340 = call <userlib>:"Wait (ms)__ogtk.vi"("error in (no error)"=w869, "milliseconds to wait"=w875) -> ("error out"=w872:errorcluster)  [unwired: 8 in, 1 out]
            n341 = call <vilib>:"Build State String with Arguments__JKI_lib_State_Machine.vi"("Arguments (\"\")"=w877, "State"="Data: Update Status") -> ("State with Arguments"=w878:string)  [unwired: 4 in]
            n342 = call <vilib>:"Add State(s) to Queue__jki_lib_state_machine.vi"("State(s) in Front (\"\")"=w878, "State(s) in (\"\")"=w888) -> ("States Out"=w887:string)  [unwired: 13 in]
          }
          frame "Sequence: Check Targets Match" {
            # "F = repeat this state. wait\nT = go to next state. don't wait"
            n343 = Unbundle By Name(w910) -> ("Running Step"=w907:i32, "setMagnet.field"=w895:dbl, "setMagnet.field"=w894:dbl, "SMO"=w893:refnum<class "Instrument.Oxford1820.lvclass">)
            n344 = call "Read IPS PSU Targets.vi"("error in (no error)"=w889, "Instrument.Oxford1820 in"=w893) -> ("error out"=w890:errorcluster, "Target Field Rate (T/min)"=w891:dbl, "Target Field (T)"=w892:dbl)  [unwired: 6 in, 1 out]
            n345 = call "Instrument.1820.FloatApprox.vi"("y"=w892, "x"=w895) -> ("x ~ y?"=w899:bool)  [unwired: 4 in]
            n346 = call "Instrument.1820.FloatApprox.vi"("y"=w891, "x"=w894) -> ("x ~ y?"=w898:bool)  [unwired: 4 in]
            n347 = And(x=w899, y=w898) -> (x .and. y?=w897:bool)
            n348 = Increment(x=w907) -> (x+1=w908:i32)
            n349 = Select(t=w908, s=w897, f=w907) -> (s? t:f=w906:i32)
            n350 = Select(t=u32 0, s=w897, f=u32 500 ("milliseconds to wait")) -> (s? t:f=w901:u32)
            n351 = Bundle By Name(cluster=w910, "Running Step"=w906) -> (w909:T12)
            n352 = call <userlib>:"Wait (ms)__ogtk.vi"("error in (no error)"=w890, "milliseconds to wait"=w901) -> ("error out"=w903:errorcluster)  [unwired: 8 in, 1 out]
            n353 = call <vilib>:"Build State String with Arguments__JKI_lib_State_Machine.vi"("Arguments (\"\")"=w904, "State"="Data: Update Status") -> ("State with Arguments"=w896:string)  [unwired: 4 in]
            n354 = call <vilib>:"Add State(s) to Queue__jki_lib_state_machine.vi"("State(s) in Front (\"\")"=w896, "State(s) in (\"\")"=w913) -> ("States Out"=w912:string)  [unwired: 13 in]
          }
        }
      }
    }
    frame Error {
    }
  }
  n355 = call-parent "Process.vi"("error in"=w5, "Instrument"=w4) -> ("error out"=w2:errorcluster, "Instrument out"=→"Instrument.Example out":refnum<class "Instrument.Oxford1820.lvclass">)  [unwired: 8 in]
  n356 = Merge Errors(w2, w1) -> (→"error out":errorcluster)
